vi "运维调试_采配水.vi"() -> ()   [LabVIEW 2016, in "PLC.lvlib"]
uses:
  PLC.lvlib
  <vilib>/Plasmionique/MB Master/MB_Master/MB_Master.lvclass
  <vilib>/Utility/miscctls.llb/LVPointTypeDef.ctl
  <vilib>/Plasmionique/MB Master/MB_Master_Serial/MB_Master_Serial.lvclass
  C:/Program Files (x86)/National Instruments/LabVIEW 2016/vi.lib/Plasmionique/MB Master/MB_Master/MB_Master.lvclass
  <vilib>/Instr/_visa.llb/VISA Configure Serial Port (Instr).vi
  <vilib>/Plasmionique/MB Master/MB Master.lvlib
panel:
  in  "看门狗启用":bool
  out "R123":i16 caption="看门狗设置"
  out "R56":i16 caption="看门狗计时器"
  in  "释放串口":bool
  out "R122":i16 caption="二级自来水清洗时间"
  out "R121":i16 caption="一级自来水清洗时间"
  out "R120":i16 caption="过滤自来水清洗时间"
  out "清洗次数":u16
  out "R119":i16 caption="多参数启动延时"
  out "当前启动泵号":u16(ring) items=["1号泵", "2号泵"]
  out "R116":i16 caption="储水时间"
  in  "R113":u16(ring) caption="水箱储水水体" items=["自来水", "水样"]
  out "R112":i16 caption="二级水样池进样超时"
  in  "R111":u16(ring) caption="采配水型号" items=["常规版本", "高配版本"]
  out "数值 19":dbl
  out "数值 18":dbl
  out "数值 17":dbl
  out "数值 16":dbl
  out "数值 15":dbl
  out "数值 14":dbl
  out "数值 13":dbl
  out "数值 12":dbl
  out "数值 11":dbl
  out "数值 10":dbl
  out "数值 9":dbl
  out "数值 8":dbl
  out "数值 7":dbl
  out "数值 6":dbl
  out "数值 5":dbl
  out "数值 4":dbl
  out "数值 3":dbl
  out "数值 2":dbl
  out "数值":dbl
  in  "R118":u16(ring) caption="是否启用质控" items=["不启用质控", "启用质控"]
  out "压力传感器":dbl format="%#.2f"
  out "R110":i16 caption="过滤装置排液时间"
  in  "M4":bool
  in  "M3":bool
  in  "V13":bool
  in  "V12":bool
  in  "V1-R":bool
  in  "V1-G":bool
  in  "V11":bool
  in  "V10":bool
  in  "V9":bool
  in  "V8":bool
  in  "V7-R":bool
  in  "V7-G":bool
  out "X2":bool caption="X1"
  out "采配水版本号":string
  out "R117":i16 caption="清洗频次设定"
  out "通讯故障":bool
  in  "R100":u16(ring) caption="采水泵工作模式" items=["泵1单泵单管路", "泵2单泵单管路", "潜水泵双泵双管路", "自吸泵双泵双管路"]
  out "X11":bool caption="自来水检测_WA"
  out "X10":bool caption="废液报警_WLA"
  out "X9":bool caption="泵2过载报警_KM2"
  out "X8":bool caption="泵1过载报警_KM1"
  out "X7":bool caption="断电检测_DD"
  out "X6":bool caption="门禁开关_MJ"
  out "X5":bool caption="烟雾检测_YW"
  out "X4":bool caption="浸水检测_SJ"
  out "X3":bool caption="水流开关_JY"
  out "X1":bool
  out "X0":bool caption="采样池液位开关_YE1"
  out "R109":i16 caption="外部反冲洗时间"
  out "集成报警信息":string
  out "R108":i16 caption="进样超时时间"
  out "R107":i16 caption="进气时间"
  out "R106":i16 caption="排液时间"
  out "R105":i16 caption="配水时间"
  out "R104":i16 caption="过滤次数"
  out "R103":i16 caption="过滤配水时间"
  out "R102":i16 caption="静置沉淀时间"
  out "R101":i16 caption="管路润洗时间"
  out "R2":i16
  out "R1":i16
  out "多列列表框":i32(listbox)
  in  "V6":bool
  in  "V5":bool
  in  "V4":bool
  in  "V3":bool
  in  "V2":bool
  in  "M2":bool
  in  "M1":bool
  in  "返回":bool
  in  "参数设置":bool
  in  "单步启动":bool
  in  "启动":bool
  in  "停止":bool
  # "流程计时："
  # "s"
  # "压力传感器："
  # "MPa"
  # "二级液位开关低_Y2FD"
  # "二级液位开关高_YF2H"
  # "看门狗设置"
  # "S"
  # "S"
  # "S"
  # "S"
  # "S"
  # "S"
  # "S"
  # "S"
  # "次"
  # "S"
  # "S"
  # "S"
  # "S"
  # "S"
  # "S"
  # "单步计时："
  # "s"
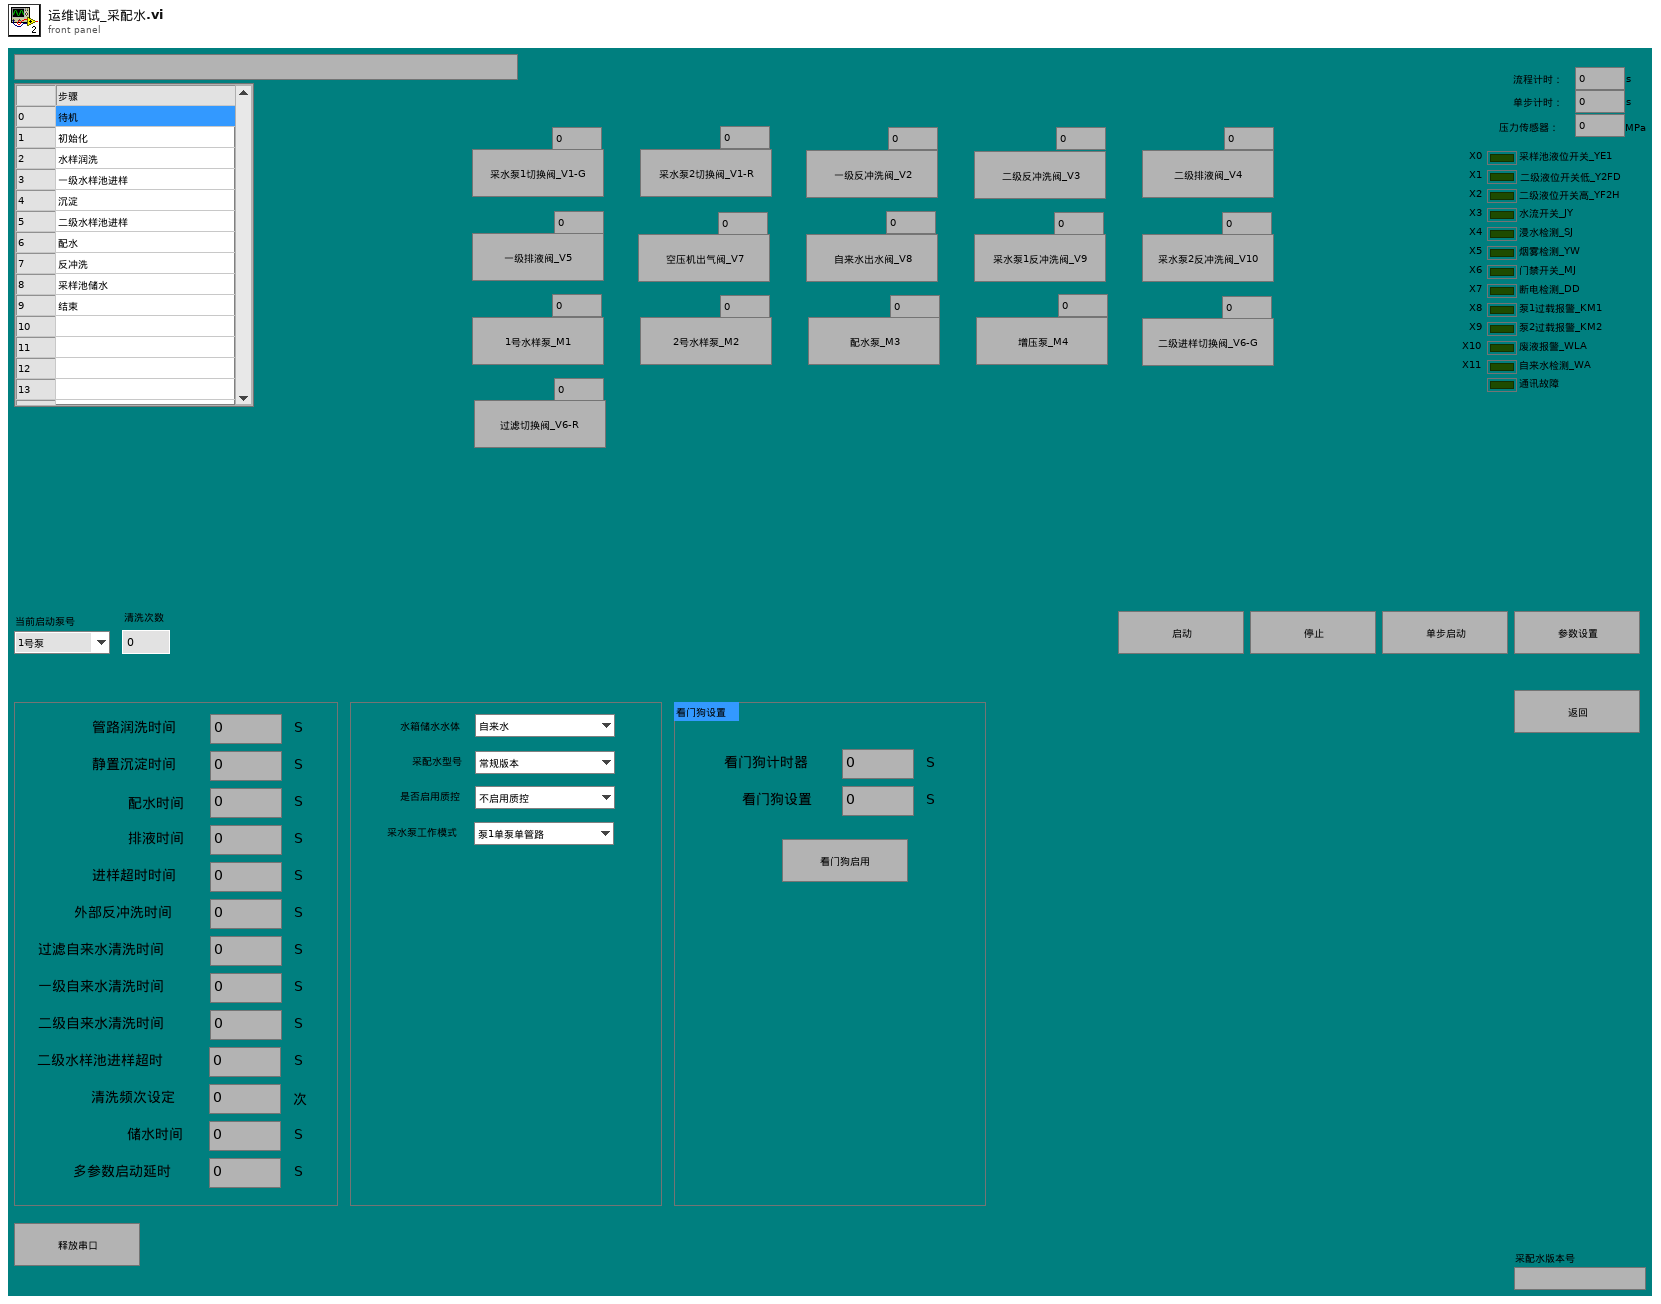
[diagram p1: front panel]
types:
  T1 = typedef "LVPointTypeDef.ctl" = cluster{"Horizontal":i16, "Vertical":i16}
  T2 = cluster{"命令":string, "数据":cluster{"starting address":u16, "holding register value":u16}}
  T3 = cluster{"时间标识":timestamp, "设备":string, "日志信息":string}
  T4 = cluster{"R0":i16, "R1":i16, "R2":i16, "R3":i16, "R4":i16, "R5":i16, "R6":i16, "R7":i16, "R8":i16, "R9":i16, "R10":i16, "R11":i16, "R12":i16, "R13":i16, "R14":i16, "R15":i16, "R16":i16, "R17":i16, "R18":i16, "R19":i16, "R20":i16, "R21":i16, "R22":i16, "R23":i16, "R24":i16, "R25":i16, "R26":i16, "R27":i16, "R28":i16, "R29":i16, "R30":i16, "R31":i16, "R32":i16, "R33":i16, "R34":i16, "R35":i16, "R36":i16, "R37":i16, "R38":i16, "R39":i16, "R40":i16, "R41":i16, "R42":i16, "R43":i16, "R44":i16, "R45":i16, "R46":i16, "R47":i16, "R48":i16, "R49":i16, "R50":i16, "R51":i16, "R52":i16, "R53":i16, "R54":i16, "R55":i16, "R56":i16}
  T5 = cluster{"seconds since 1Jan1904":timestamp, "table输入":string, string, "table输入":string}
  T6 = cluster{"时间标识":timestamp, "设备":string, "日志信息":string, "流程参数":string}
  T7 = cluster{"命令":string, cluster{"starting address":u16, "holding register value":u16}}
  T8 = cluster{"CODCr":cluster{"启动测量模式":cluster{"测量模式":enum16{"水样测量", "标样核查", "零点核查", "跨度核查", "空白测试", "加标回收", "平行样", "校零", "校标"}}, "确定按钮":bool}, "参数启用":cluster{"多参数":bool, "CODMn":bool, "总磷总氮":bool, "氨氮":bool, "CODcr":bool}}
  T9 = enum16{"水样测量", "标样核查", "零点核查", "跨度核查", "空白测试", "加标回收", "平行样", "校零", "校标"}
  T10 = cluster{"命令":string, "数据":cluster{"starting address":u16, "holding register values":u16[]}}
  T11 = cluster{"命令":string, "data":cluster{"starting address":u16, "coil values":bool[]}}
  T12 = cluster{"多参数":bool, "CODMn":bool, "总磷总氮":bool, "氨氮":bool, "CODcr":bool}
  T13 = enum32{"Bad", "Idle", "Run top level", "Running"}
  T14 = cluster{"baud rate (bps)":u32, "stop bits":u16, "parity":u16, "flow control":u16, "timeout":u32, "retries":i32}
  T15 = cluster{"starting address":u16, "holding register values":u16[]}
  T16 = cluster{"starting address":u16, "holding register value":u16}
  T17 = cluster{"starting address":u16, "coil values":bool[]}
  T18 = cluster{"Registers[0]":u16, "Registers[1]":u16, "Registers[2]":u16, "Registers[3]":u16, "Registers[4]":u16, "Registers[5]":u16, "Registers[6]":u16, "Registers[7]":u16, "Registers[8]":u16, "Registers[9]":u16, "Registers[10]":u16, "Registers[11]":u16, "Registers[12]":u16, "Registers[13]":u16, "Registers[14]":u16, "Registers[15]":u16, "Registers[16]":u16, "Registers[17]":u16, "Registers[18]":u16, "Registers[19]":u16, "Registers[20]":u16, "Registers[21]":u16, "Registers[22]":u16, "Registers[23]":u16, "Registers[24]":u16, "Registers[25]":u16, "Registers[26]":u16, "Registers[27]":u16, "Registers[28]":u16, "Registers[29]":u16, "Registers[30]":u16, "Registers[31]":u16, "Registers[32]":u16, "Registers[33]":u16, "Registers[34]":u16, "Registers[35]":u16, "Registers[36]":u16, "Registers[37]":u16, "Registers[38]":u16, "Registers[39]":u16, "Registers[40]":u16, "Registers[41]":u16, "Registers[42]":u16, "Registers[43]":u16, "Registers[44]":u16, "Registers[45]":u16, "Registers[46]":u16, "Registers[47]":u16, "Registers[48]":u16, "Registers[49]":u16, "Registers[50]":u16, "Registers[51]":u16, "Registers[52]":u16, "Registers[53]":u16, "Registers[54]":u16, "Registers[55]":u16, "Registers[56]":u16}
  T19 = cluster{"Registers[0]":u16, "Registers[1]":u16, "Registers[2]":u16, "Registers[3]":u16, "Registers[4]":u16, "Registers[5]":u16}
  T20 = cluster{"Registers[0]":u16, "Registers[1]":u16, "Registers[2]":u16, "Registers[3]":u16, "Registers[4]":u16, "Registers[5]":u16, "Registers[6]":u16, "Registers[7]":u16, "Registers[8]":u16, "Registers[9]":u16, "Registers[10]":u16, "Registers[11]":u16, "Registers[12]":u16, "Registers[13]":u16, "Registers[14]":u16, "Registers[15]":u16, "Registers[16]":u16, "Registers[17]":u16, "Registers[18]":u16, "Registers[19]":u16, "Registers[20]":u16, "Registers[21]":u16, "Registers[22]":u16, "Registers[23]":u16}
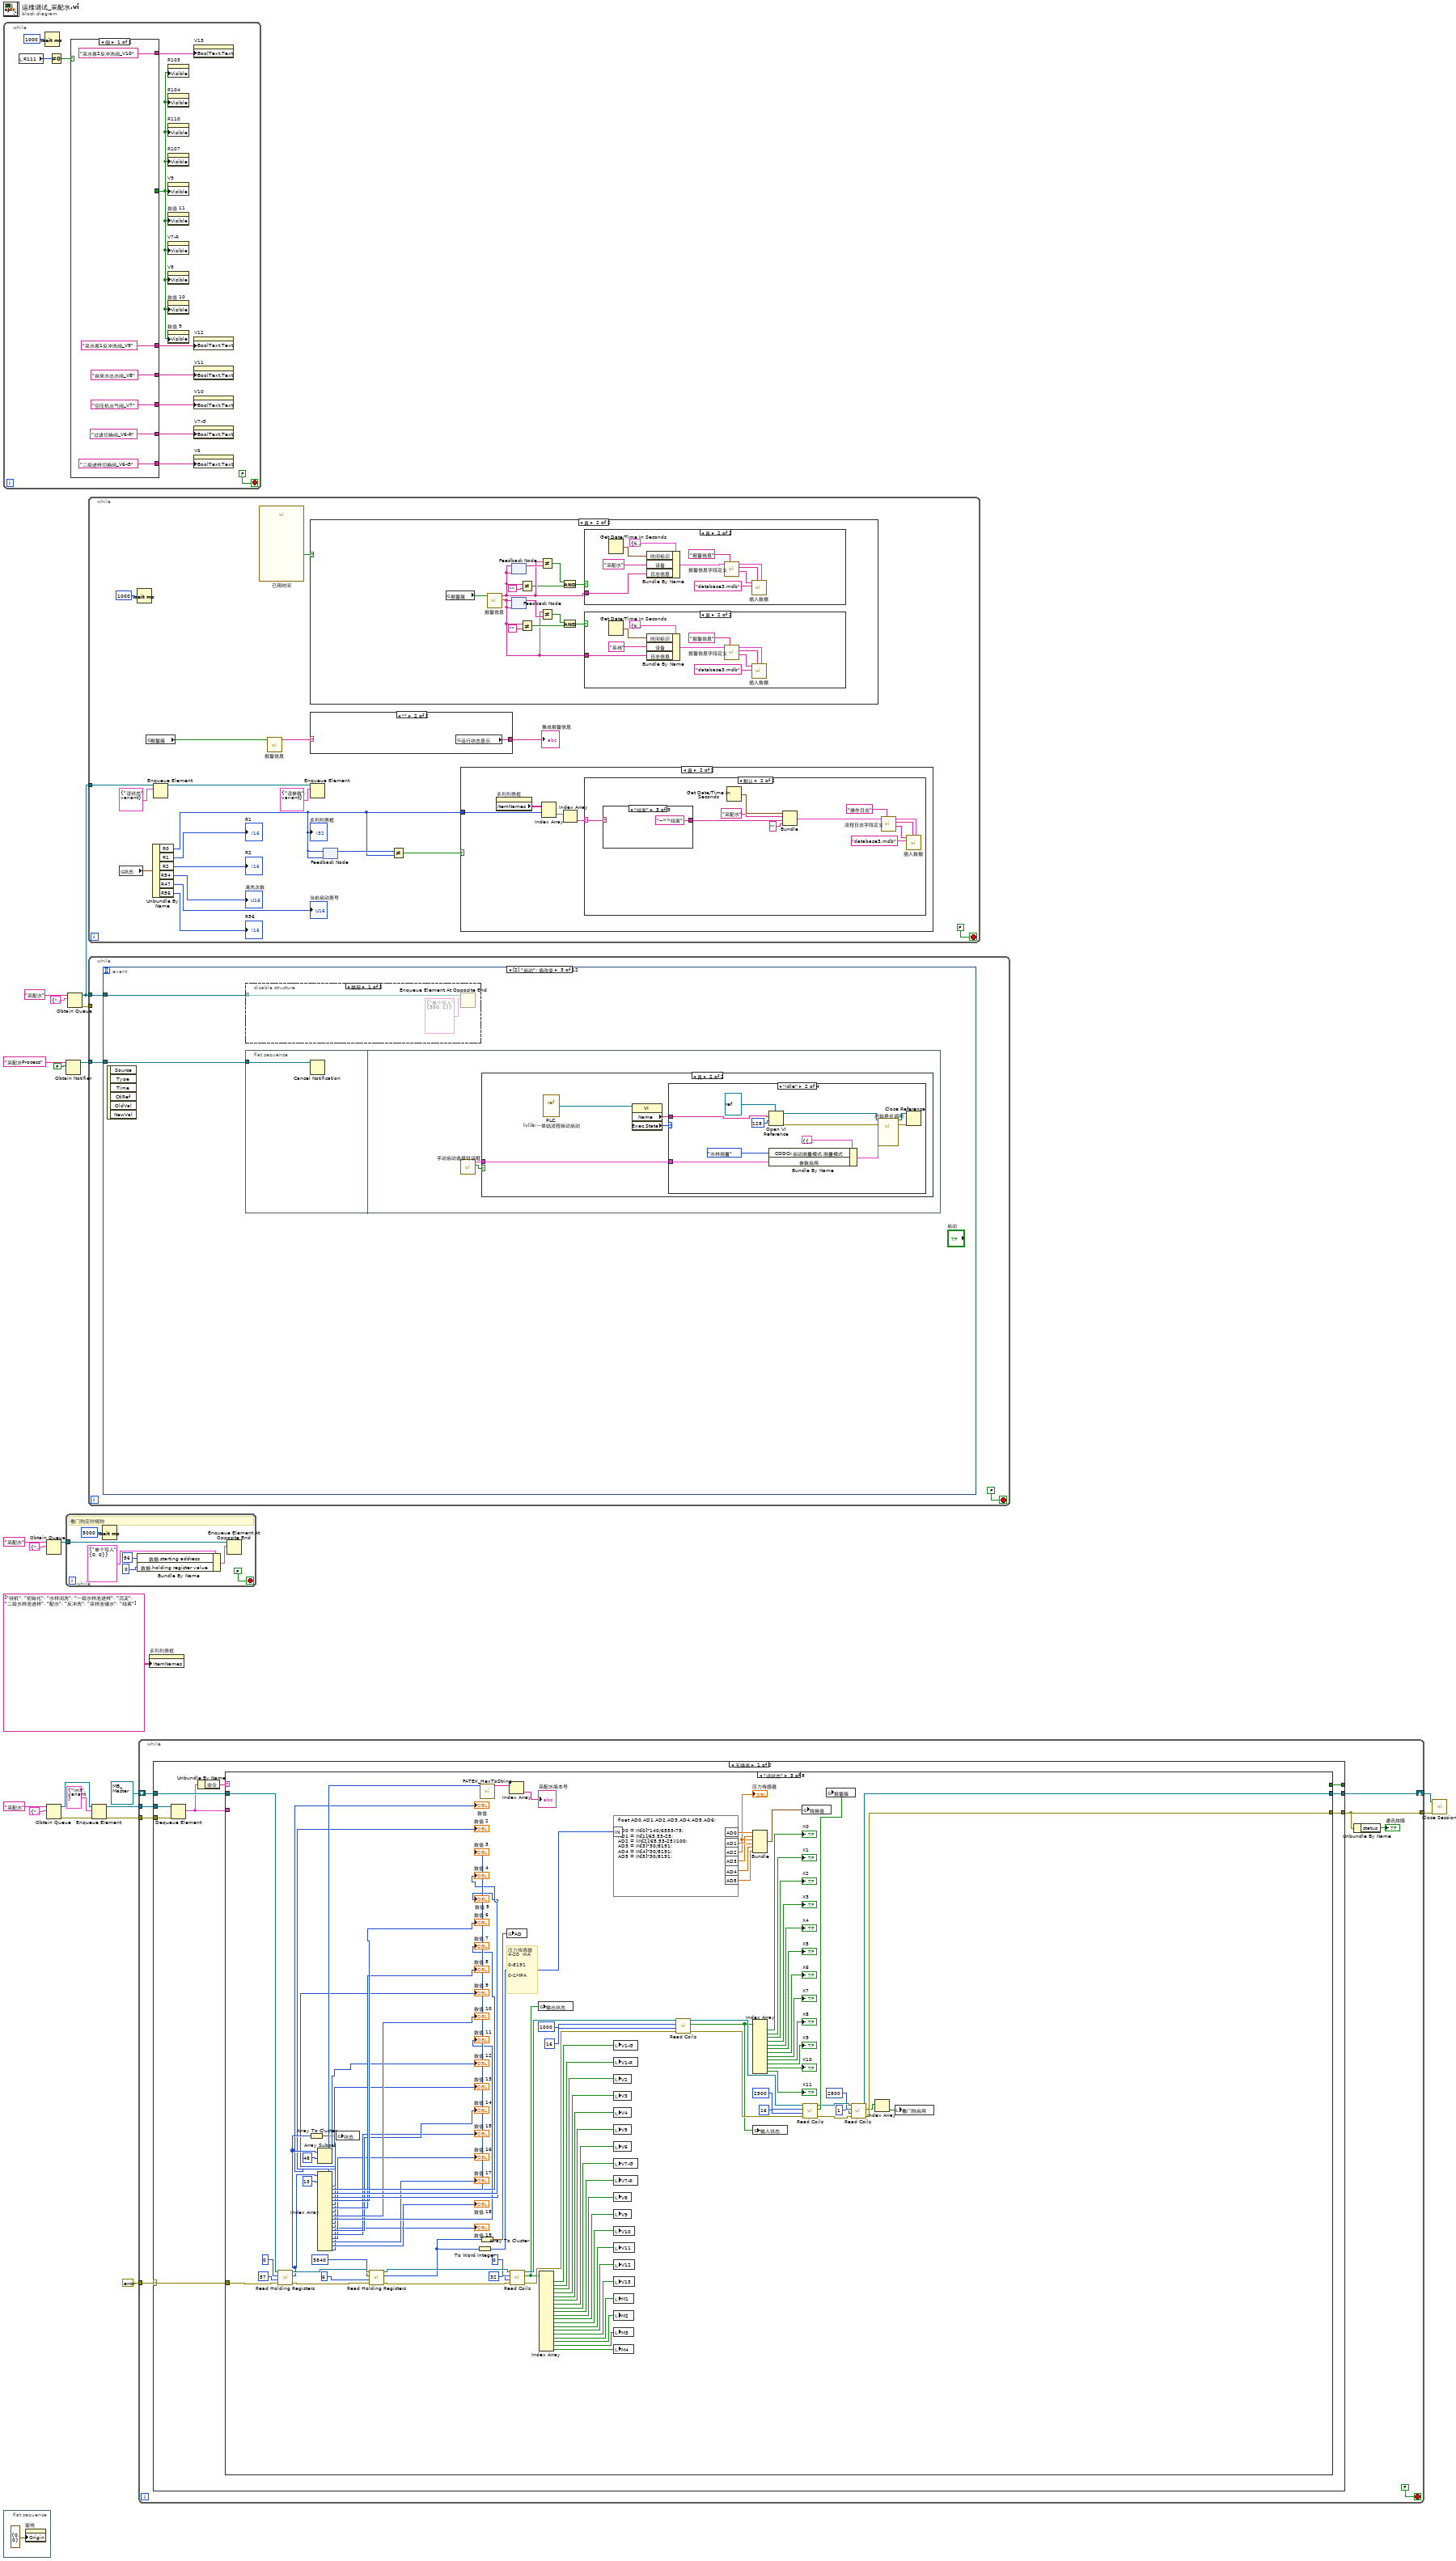
[diagram p0: block diagram]
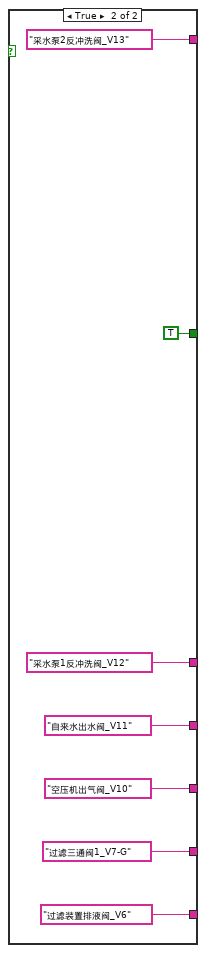
[diagram p2: hidden frame]
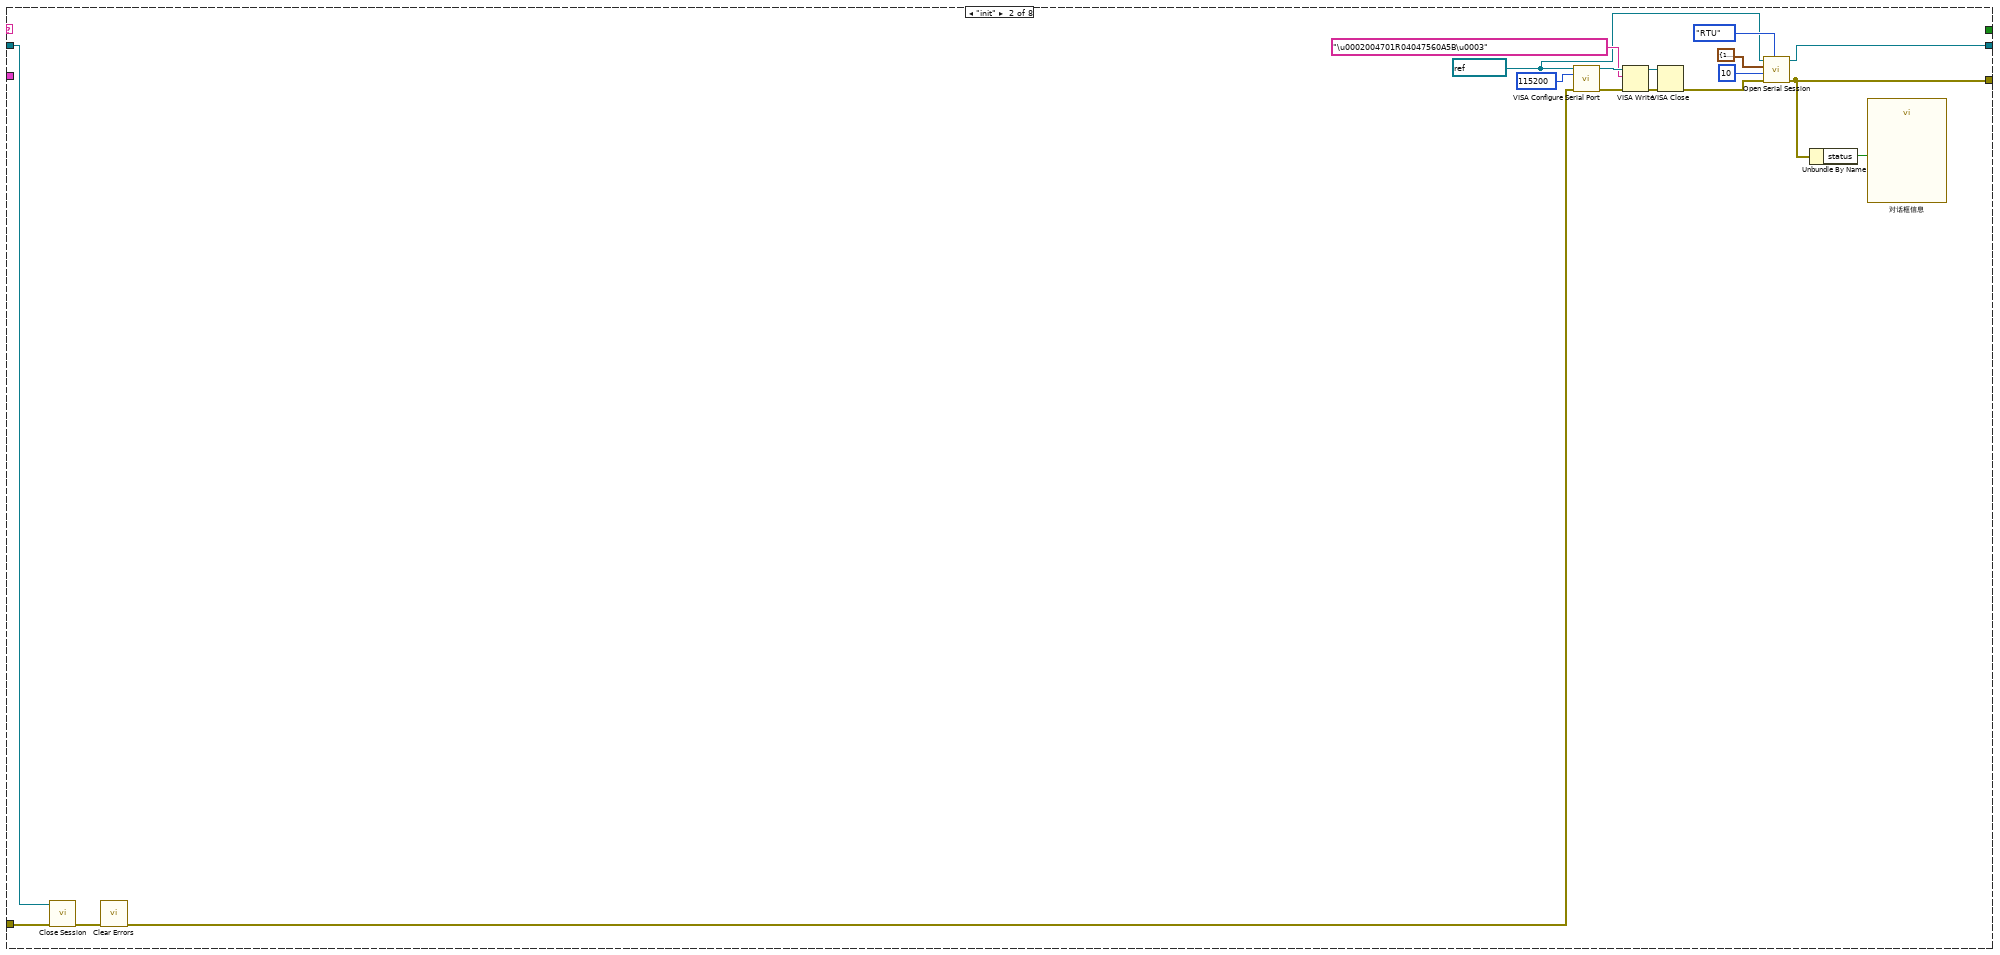
[diagram p4: hidden frame]
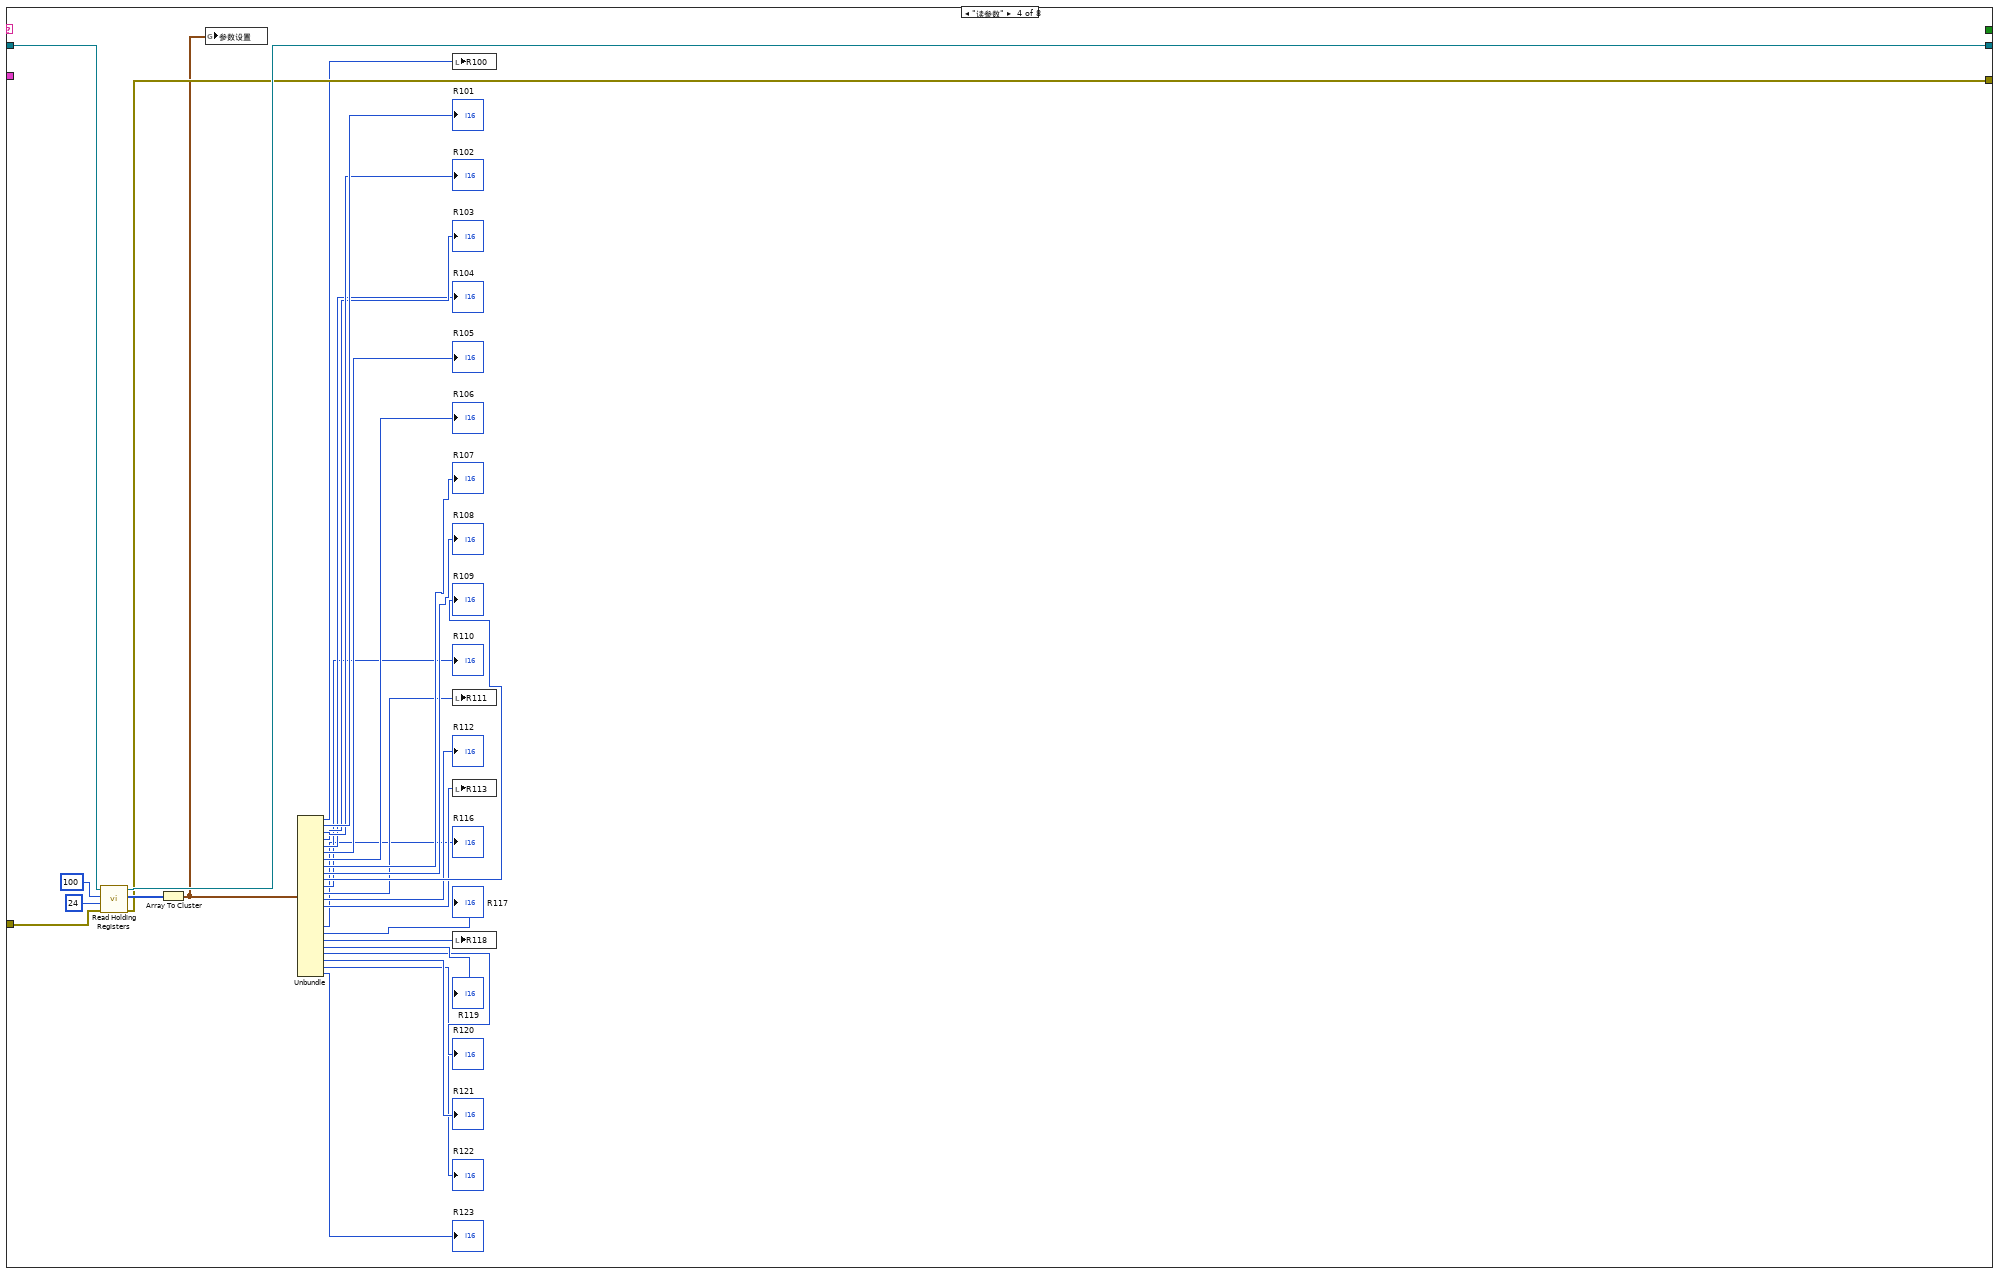
[diagram p5: hidden frame]
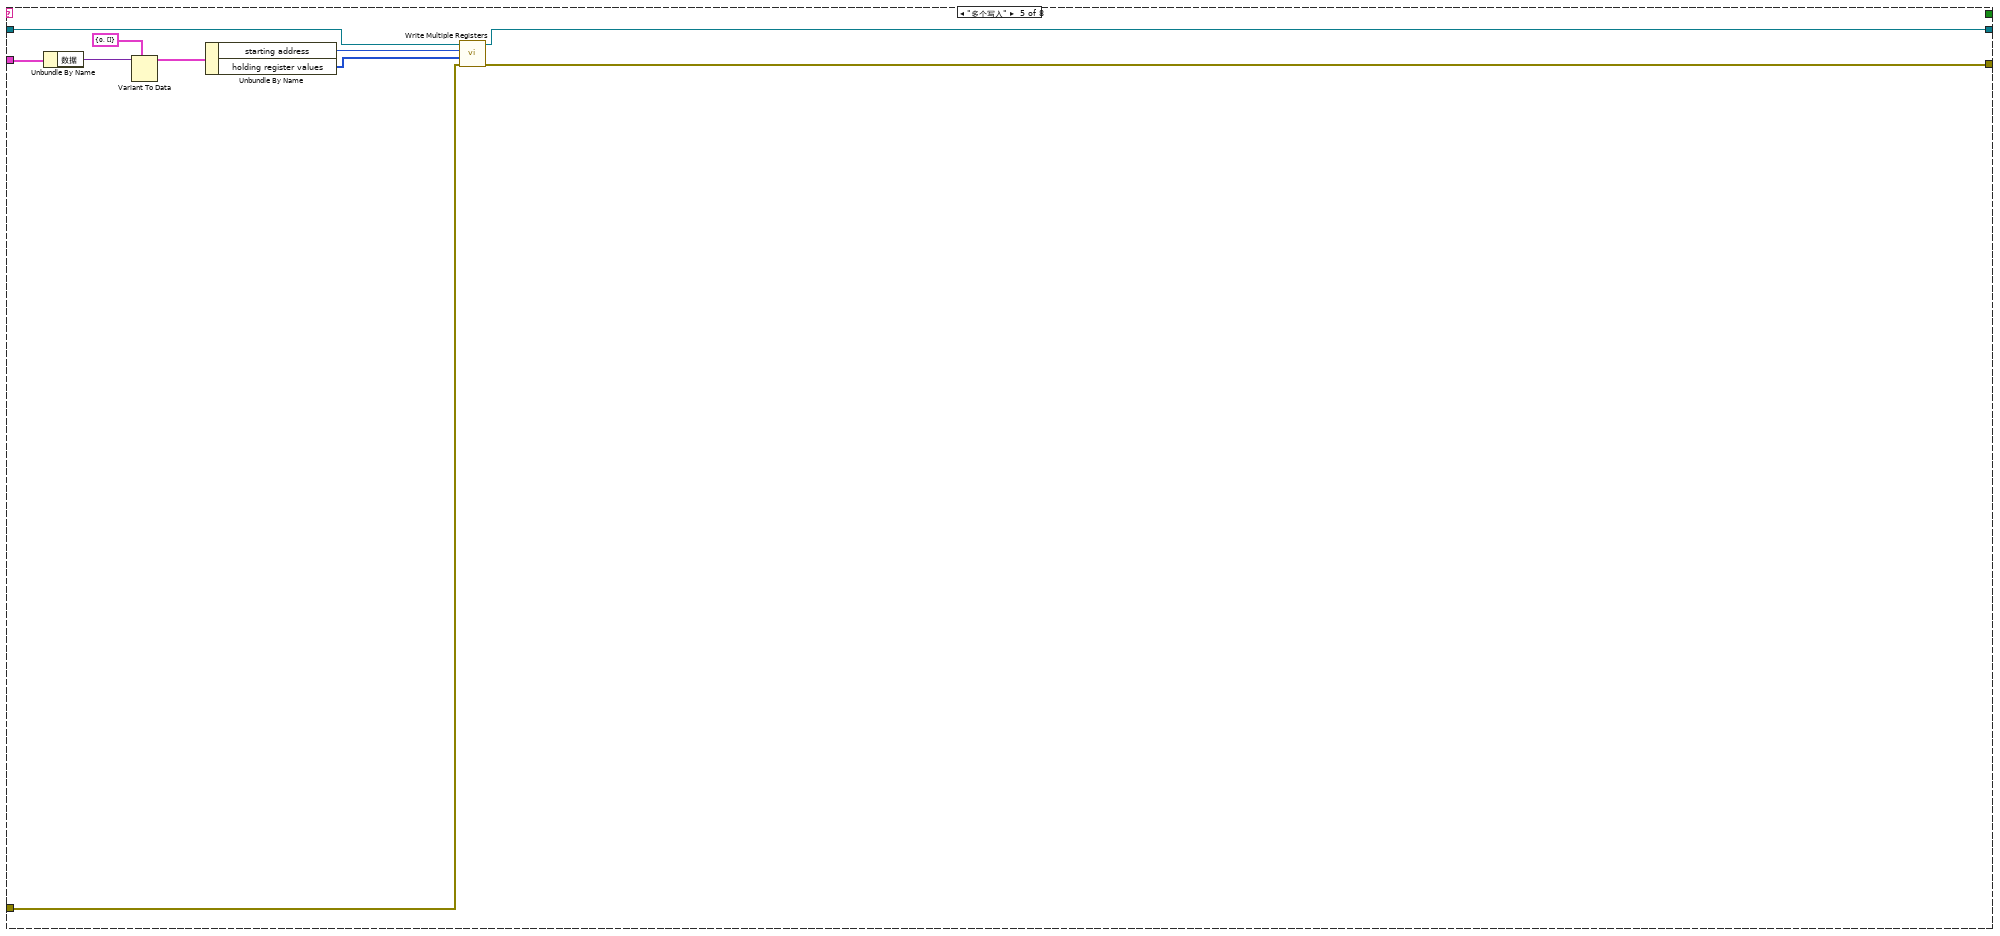
[diagram p6: hidden frame]
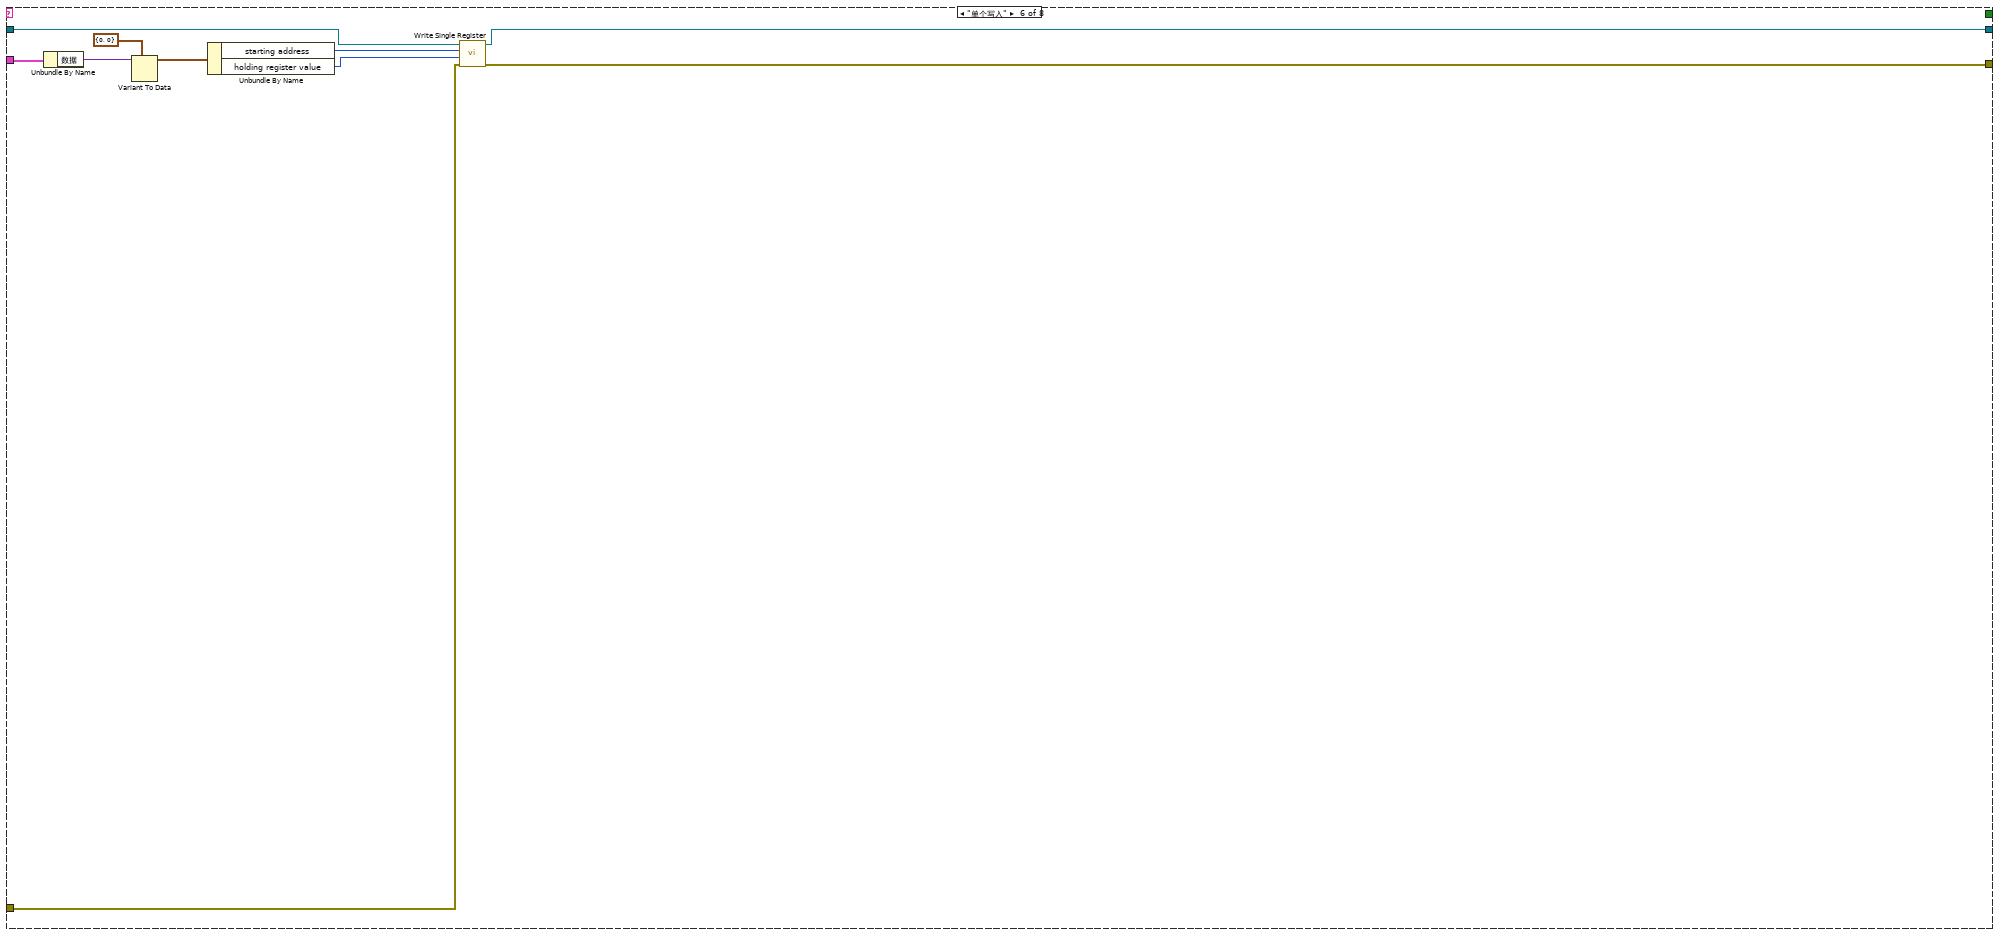
[diagram p7: hidden frame]
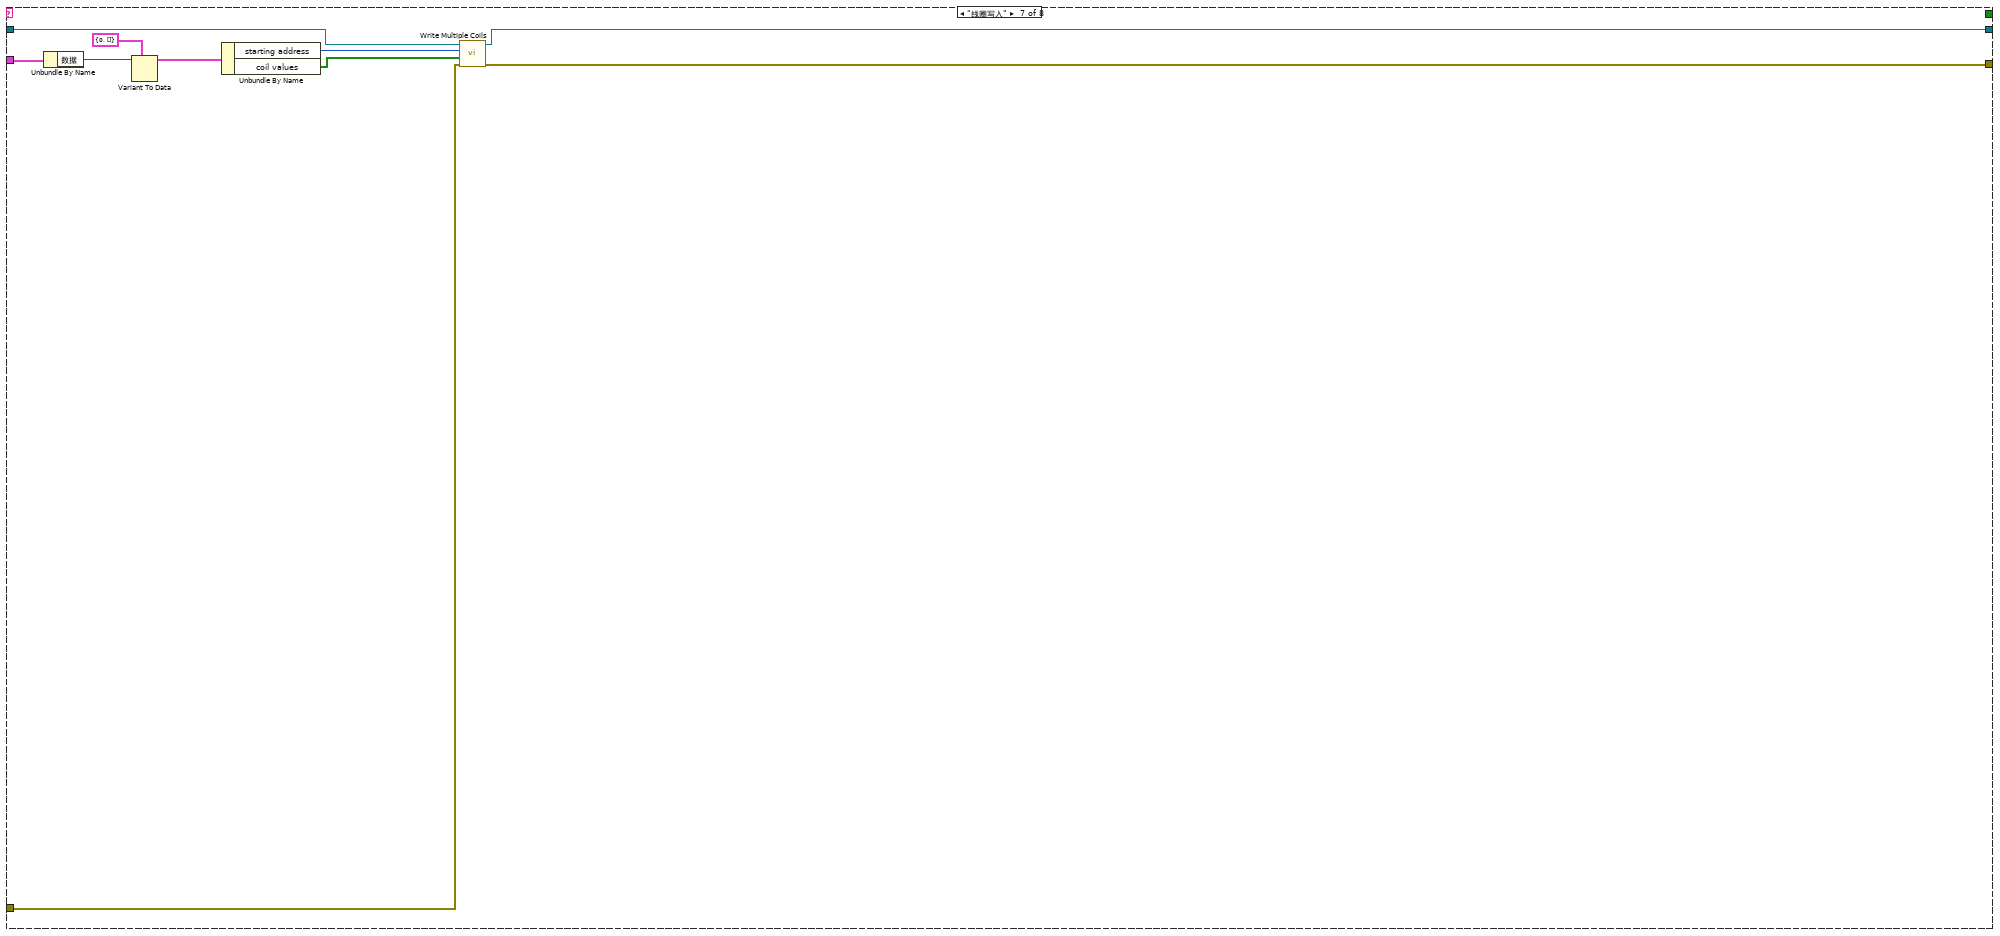
[diagram p8: hidden frame]
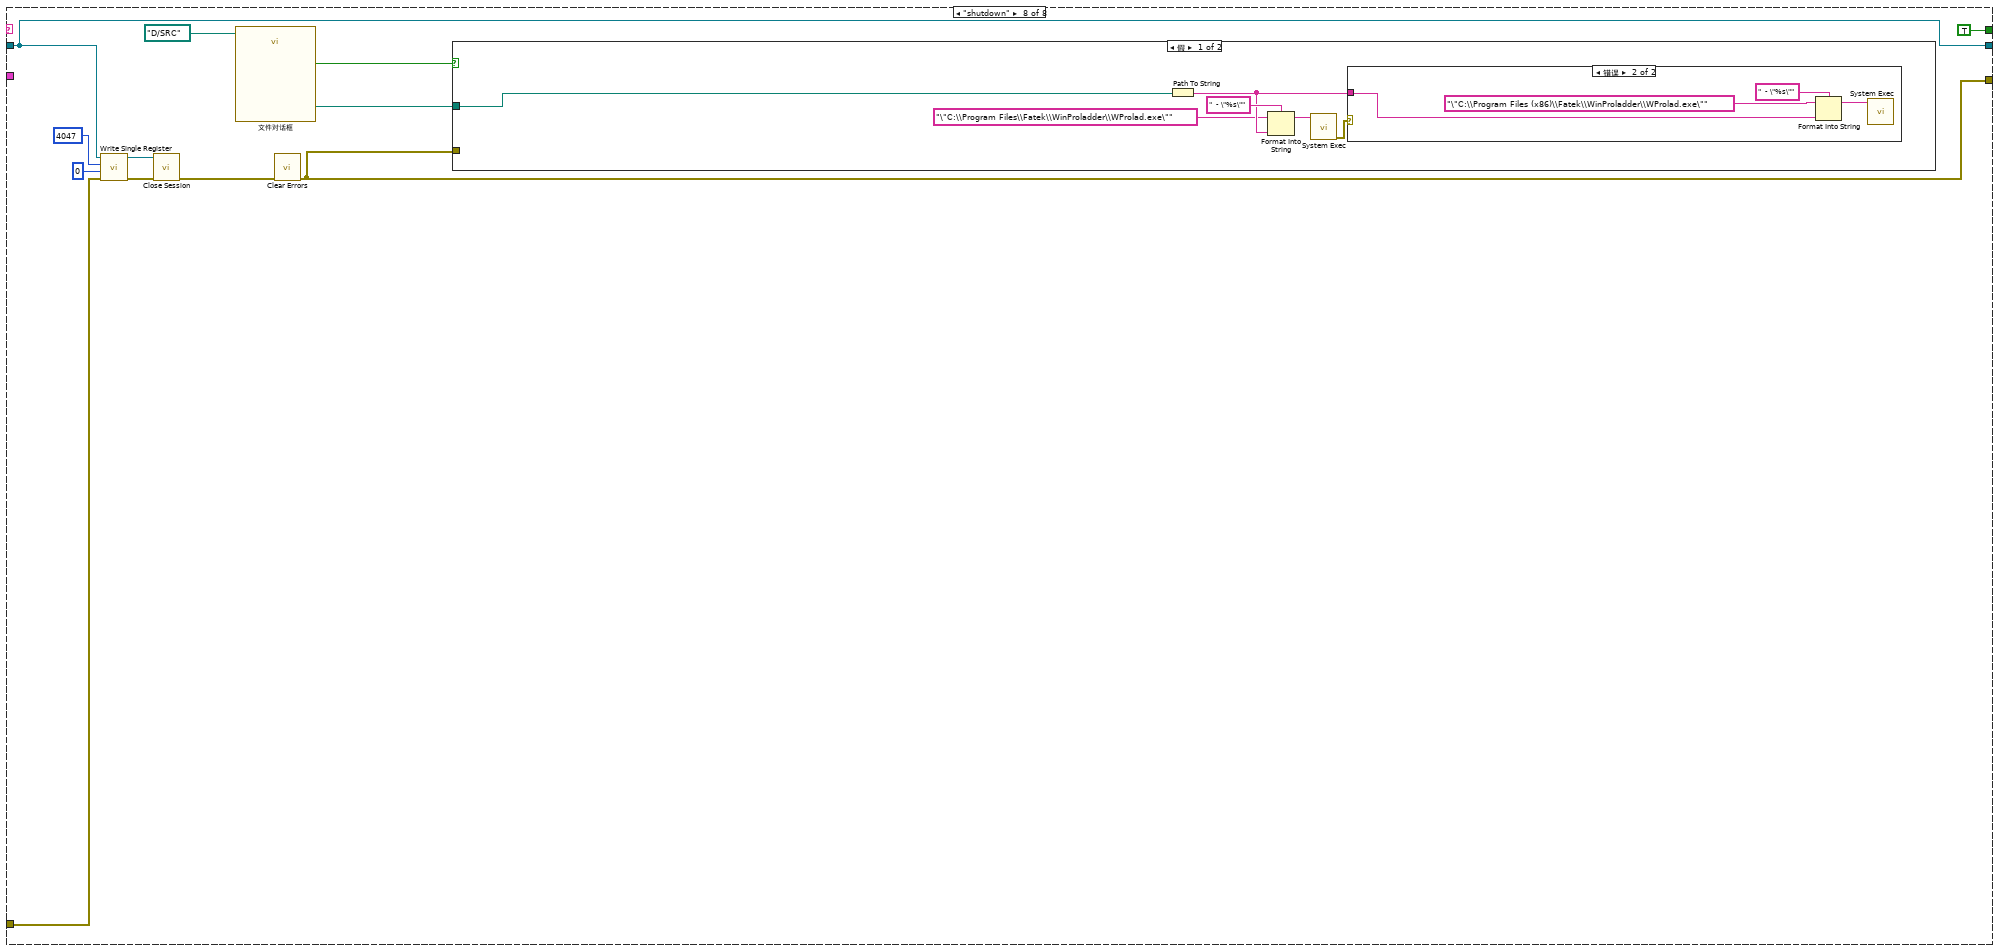
[diagram p9: hidden frame]
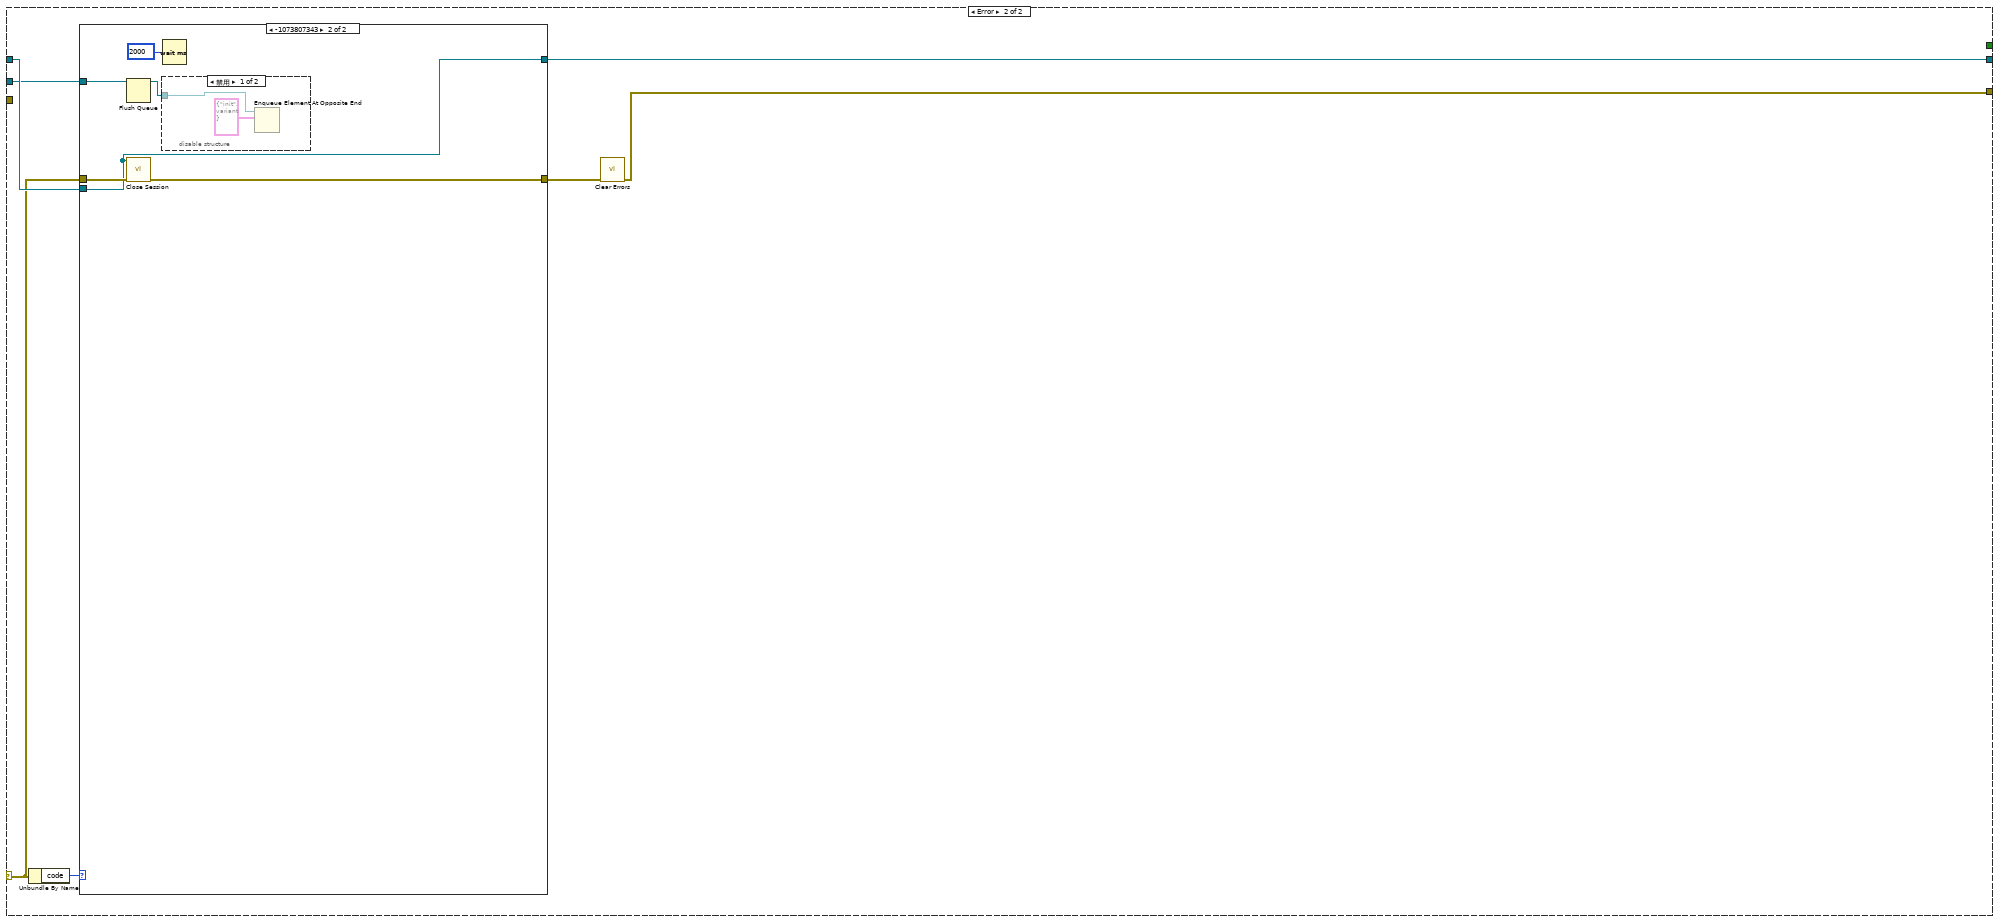
[diagram p12: hidden frame]
diagram:
  n1 = while {
    stop <- FALSE stop-if-true
    n2 = local read "R111"() -> (w32:u16)
    n3 = Wait (ms)(milliseconds to wait=u32 1000 ("等待时间（毫秒）")) -> ()  [unwired: 1 out]
    n4 = Not Equal To 0?(x=w32) -> (x != 0?=w31:bool)
    n5 = case shown="假" w31 {
      tunnel: [_ TRUE ("可见")] -> w30
      tunnel: ["二级进样切换阀_V6-G" ("布尔文本.文本") "过滤装置排液阀_V6" ("布尔文本.文本")] -> w28
      tunnel: ["过滤切换阀_V6-R" ("布尔文本.文本") "过滤三通阀1_V7-G" ("布尔文本.文本")] -> w27
      tunnel: ["空压机出气阀_V7" ("布尔文本.文本") "空压机出气阀_V10" ("布尔文本.文本")] -> w26
      tunnel: ["自来水出水阀_V8" ("布尔文本.文本") "自来水出水阀_V11" ("布尔文本.文本")] -> w25
      tunnel: ["采水泵1反冲洗阀_V9" ("布尔文本.文本") "采水泵1反冲洗阀_V12" ("布尔文本.文本")] -> w24
      tunnel: ["采水泵2反冲洗阀_V10" ("布尔文本.文本") "采水泵2反冲洗阀_V13" ("布尔文本.文本")] -> w23
      frame False {
      }
      frame True {
      }
    }
    n6 = property on="R103" class="DigNum (严格)"("Visible"=w30) -> ()  [unwired: 2 in, 2 out]
    n7 = property on="R104" class="DigNum (严格)"("Visible"=w30) -> ()  [unwired: 2 in, 2 out]
    n8 = property on="R110" class="DigNum (严格)"("Visible"=w30) -> ()  [unwired: 2 in, 2 out]
    n9 = property on="R107" class="DigNum (严格)"("Visible"=w30) -> ()  [unwired: 2 in, 2 out]
    n10 = property on="V9" class="Bool (严格)"("Visible"=w30) -> ()  [unwired: 2 in, 2 out]
    n11 = property on="数值 11" class="DigNum (严格)"("Visible"=w30) -> ()  [unwired: 2 in, 2 out]
    n12 = property on="V7-R" class="Bool (严格)"("Visible"=w30) -> ()  [unwired: 2 in, 2 out]
    n13 = property on="V8" class="Bool (严格)"("Visible"=w30) -> ()  [unwired: 2 in, 2 out]
    n14 = property on="数值 10" class="DigNum (严格)"("Visible"=w30) -> ()  [unwired: 2 in, 2 out]
    n15 = property on="数值 9" class="DigNum (严格)"("Visible"=w30) -> ()  [unwired: 2 in, 2 out]
    n16 = property on="V13" class="Bool (严格)"("BoolText.Text"=w23) -> ()  [unwired: 2 in, 2 out]
    n17 = property on="V12" class="Bool (严格)"("BoolText.Text"=w24) -> ()  [unwired: 2 in, 2 out]
    n18 = property on="V11" class="Bool (严格)"("BoolText.Text"=w25) -> ()  [unwired: 2 in, 2 out]
    n19 = property on="V10" class="Bool (严格)"("BoolText.Text"=w26) -> ()  [unwired: 2 in, 2 out]
    n20 = property on="V7-G" class="Bool (严格)"("BoolText.Text"=w27) -> ()  [unwired: 2 in, 2 out]
    n21 = property on="V6" class="Bool (严格)"("BoolText.Text"=w28) -> ()  [unwired: 2 in, 2 out]
  }
  n22 = flat-sequence {
    frame #0 {
      n23 = property on="窗格" class="Pane"("Origin"=T1 {"Horizontal"=0, "Vertical"=0} ("原点")) -> ()  [unwired: 2 in, 2 out]
    }
  }
  n24 = Obtain Queue(name (unnamed)="采配水" ("名称（未命名）"), element data type=cluster{"命令":string, "数据":variant} {"命令"="", "数据"=variant}) -> (queue out=w1:refnum<queue>)  [unwired: 3 in, 2 out]
  n25 = Obtain Queue(name (unnamed)="采配水" ("名称（未命名）"), element data type=cluster{"命令":string, "数据":variant} {"命令"="", "数据"=variant}) -> (queue out=w12:refnum<queue>, error out=w11:errorcluster)  [unwired: 3 in, 1 out]
  n26 = Obtain Notifier(name (unnamed)="采配水Process" ("名称（未命名）"), notification data type=FALSE) -> (notifier out=w15:refnum<notifier>)  [unwired: 2 in, 2 out]
  n27 = while {
    tunnel: w1 -> [w52]
    stop <- FALSE stop-if-true
    # "看门狗定时喂狗"
    n28 = Wait (ms)(milliseconds to wait=u32 5000 ("等待时间（毫秒）")) -> ()  [unwired: 1 out]
    n29 = Bundle By Name(cluster=T2 {"命令"="单个写入", "数据"={"starting address"=0, "holding register value"=0}} ("元素"), "数据.starting address"=u16 56, "数据.holding register value"=u16 0) -> (w53:T2)
    n30 = Enqueue Element At Opposite End(queue=w52, element=w53) -> ()  [unwired: 2 in, 3 out]
  }
  n31 = Obtain Queue(name (unnamed)="采配水" ("名称（未命名）"), element data type=cluster{"命令":string, "数据":variant} {"命令"="", "数据"=variant}) -> (queue out=w19:refnum<queue>, error out=w20:errorcluster)  [unwired: 3 in, 1 out]
  n32 = while {
    tunnel: w19 -> [w72]
    stop <- FALSE stop-if-true
    n33 = global read "采配水全局变量.vi" "状态"() -> (w70:T4)
    n34 = Wait (ms)(milliseconds to wait=u32 1000 ("等待时间（毫秒）")) -> ()  [unwired: 1 out]
    n35 = global read "采配水全局变量.vi" "报警簇"() -> (w66:bool[])
    n36 = Unbundle By Name(w70) -> ("R0"=w59:i16, "R1"=→"R1":i16, "R2"=→"R2":i16, "R54"=→"清洗次数":i16, "R47"=→"当前启动泵号":i16, "R56"=→"R56":i16)
    "多列列表框" <- w59
    n37 = Enqueue Element(queue=w72, element=cluster{"命令":string, "数据":variant} {"命令"="读状态", "数据"=variant} ("元素")) -> (queue out=w61:refnum<queue>)  [unwired: 2 in, 2 out]
    n38 = call "已用时间"() -> ("Time has Elapsed"=w64:bool)  [unwired: 12 in, 7 out]
    n39 = call "报警信息.vi"("报警簇"=w66) -> ("采配水报警信息"=w58:string)  [unwired: 9 in, 1 out]
    n40 = case shown="真" w64 {
      frame False {
      }
      frame True {
        n41 = global read "采配水全局变量.vi" "报警簇"() -> (w86:bool[])
        n42 = call "报警信息.vi"("报警簇"=w86) -> ("系统报警信息"=w75:string, "采配水报警信息"=w82:string)  [unwired: 9 in]
        n43 = feedback #1(w82) -> (w85:string)
        n44 = feedback-in #1(w82) -> ()
        n45 = feedback #2(w75) -> (w76:string)
        n46 = feedback-in #2(w75) -> ()
        n47 = Not Equal?(x=w82, y="") -> (x != y?=w80:bool)
        n48 = Not Equal?(x=w75, y="") -> (x != y?=w79:bool)
        n49 = Not Equal?(x=w82, y=w85) -> (x != y?=w84:bool)
        n50 = Not Equal?(x=w75, y=w76) -> (x != y?=w77:bool)
        n51 = And(x=w84, y=w80) -> (x .and. y?=w83:bool)
        n52 = And(x=w77, y=w79) -> (x .and. y?=w74:bool)
        n53 = case shown="真" w83 {
          tunnel: w82 -> [_ w97]
          frame False {
          }
          frame True {
            n54 = Get Date/Time In Seconds() -> (seconds since 1Jan1904=w99:timestamp)
            n55 = Bundle By Name(cluster=T3 {"时间标识"=timestamp(0 s since 1904-01-01), "设备"="", "日志信息"=""} ("data in"), "时间标识"=w99, "设备"="采配水", "日志信息"=w97) -> (w100:T3)
            n56 = call "报警信息字段定义.vi"("table输入"="报警信息", "data in"=w100) -> ("table输出"=w104:string, "columns"=w105:string[], "data out"=w106:T3)  [unwired: 7 in]
            n57 = call "插入数据.vi"("data"=w106, "columns"=w105, "database"="database3.mdb", "table"=w104) -> ()  [unwired: 7 in, 1 out]
          }
        }
        n58 = case shown="真" w74 {
          tunnel: w75 -> [_ w87]
          frame False {
          }
          frame True {
            n59 = Get Date/Time In Seconds() -> (seconds since 1Jan1904=w89:timestamp)
            n60 = Bundle By Name(cluster=T3 {"时间标识"=timestamp(0 s since 1904-01-01), "设备"="", "日志信息"=""} ("data in"), "时间标识"=w89, "设备"="系统", "日志信息"=w87) -> (w90:T3)
            n61 = call "报警信息字段定义.vi"("table输入"="报警信息", "data in"=w90) -> ("table输出"=w94:string, "columns"=w95:string[], "data out"=w96:T3)  [unwired: 7 in]
            n62 = call "插入数据.vi"("data"=w96, "columns"=w95, "database"="database3.mdb", "table"=w94) -> ()  [unwired: 7 in, 1 out]
          }
        }
      }
    }
    n63 = case shown="\"\"" w58 {
      selector: w58 -> [w107 _]
      tunnel: [w107 w108] -> w65
      frame Default {
      }
      frame "" {
        n64 = global read "采配水全局变量.vi" "运行状态显示"() -> (w108:string)
      }
    }
    "集成报警信息" <- w65
    n65 = Enqueue Element(queue=w61, element=cluster{"命令":string, "数据":variant} {"命令"="读参数", "数据"=variant} ("元素")) -> ()  [unwired: 2 in, 3 out]
    n66 = feedback-in #3(w59) -> ()
    n67 = feedback #3(w59) -> (w60:i16)
    n68 = Not Equal?(x=w60, y=w59) -> (x != y?=w67:bool)
    n69 = case shown="真" w67 {
      tunnel: w59 -> [_ w111]
      frame False {
      }
      frame True {
        n70 = property on="多列列表框" class="MCListbox (严格)"() -> ("ItemNames"=w112:string[][])  [unwired: 2 in, 2 out]
        n71 = Index Array(array=w112, index (row)=w111) -> (element=w110:string[])  [unwired: 1 in]
        n72 = Index Array(array=w110) -> (element=w109:string)  [unwired: 1 in]
        n73 = case shown="默认" w109 {
          selector: w109 -> [_ w114]
          frame "待机" {
          }
          frame Default {
            n74 = case shown="\"结束\"" w114 {
              selector: w114 -> [w124 _ _]
              tunnel: [w124 "-->>初始化" "-->>结束"] -> w113
              frame Default {
              }
              frame "初始化" {
              }
              frame "结束" {
              }
            }
            n75 = Get Date/Time In Seconds() -> (seconds since 1Jan1904=w118:timestamp)
            n76 = Bundle("seconds since 1Jan1904"=w118, "table输入"="采配水", w113, "table输入"="") -> (w116:T5)  [unwired: 1 in]
            n77 = call "流程日志字段定义.vi"("table输入"="操作日志", "data in"=w116) -> ("table输出"=w121:string, "columns"=w122:string[], "data out"=w123:T6)  [unwired: 7 in]
            n78 = call "插入数据.vi"("data"=w123, "columns"=w122, "database"="database3.mdb", "table"=w121) -> ()  [unwired: 7 in, 1 out]
          }
        }
      }
    }
  }
  n79 = while {
    tunnel: w19 -> [w128]
    tunnel: w20 -> [_]
    tunnel: w15 -> [w127]
    stop <- FALSE stop-if-true
    n80 = event shown="[2] \"启动\": 值改变" {
      selector: _ -> [_ _ _ _ _ _ _ _ _ _ _ _]
      dyn-events: _ -> [_ _ _ _ _ _ _ _ _ _ _ _]
      timeout: _ -> [_ _ _ _ _ _ _ _ _ _ _ _]
      tunnel: w128 -> [_ w132 w135 w160 w179 w189 _ _ _ w221 w224 w230]
      tunnel: w127 -> [_ w131 w134 _ _ _ _ _ _ _ _ _]
      event Timeout {
        n81 = event-data() -> ()  [unwired: 1 in, 3 out]
      }
      event "停止": Value Change {
        n82 = event-data() -> ()  [unwired: 1 in, 6 out]
        n83 = Send Notification(notification=TRUE ("通知"), notifier=w131) -> ()  [unwired: 1 in, 2 out]
        n84 = Enqueue Element At Opposite End(queue=w132, element=T7 {"命令"="单个写入", {"starting address"=300, "holding register value"=2}} ("元素")) -> ()  [unwired: 2 in, 3 out]
      }
      event "启动": Value Change {
        n85 = event-data() -> ()  [unwired: 1 in, 6 out]
        n86 = disable-structure shown="禁用" {
          disable-tunnel: w135 -> [w156 _]
          frame Disabled {
            n87 = Enqueue Element At Opposite End(queue=w156, element=T7 {"命令"="单个写入", {"starting address"=300, "holding register value"=1}} ("元素")) -> ()  [unwired: 2 in, 3 out]
          }
          frame Enabled {
          }
        }
        n88 = flat-sequence {
          tunnel: w134 -> [w136]
          frame #0 {
            n89 = Cancel Notification(0:w136) -> ()  [unwired: 1 in, 3 out]
          }
          frame #1 {
            n90 = call "手动启动选择对话框.vi"() -> ("确定"=w138:bool, "参数启用"=w137:T12)  [unwired: 10 in]
            n91 = case shown="真" w138 {
              tunnel: w137 -> [_ w139]
              frame False {
              }
              frame True {
                n92 = vi-ref "PLC.lvlib:一体站流程自动启动.vi"() -> (w142:refnum<vi>)
                n93 = property class="VI"(reference=w142) -> ("Name"=w141:string, "Exec.State"=w140:T13)  [unwired: 1 in, 2 out]
                n94 = case shown="\"Idle\"" w140 {
                  tunnel: w141 -> [_ w153 _ _]
                  tunnel: w139 -> [_ w147 _ _]
                  frame "Bad", Default {
                  }
                  frame "Idle" {
                    n95 = Bundle By Name(cluster=T8 {"CODCr"={"启动测量模式"={"测量模式"=enum."水样测量"}, "确定按钮"=FALSE}, "参数启用"={"多参数"=FALSE, "CODMn"=FALSE, "总磷总氮"=FALSE, "氨氮"=FALSE, "CODcr"=FALSE}} ("参数"), "CODCr.启动测量模式.测量模式"=T9."水样测量", "参数启用"=w147) -> (w143:T8)
                    n96 = Open VI Reference(type specifier VI Refnum (for type only)=refnum<vi> refnum, vi path=w153, options=128 ("选项")) -> (vi reference=w151:refnum<vi>, error out=w149:errorcluster)  [unwired: 3 in]
                    n97 = call-by-ref "开始异步调用"(reference=w151, error in=w149, "参数"=w143) -> (reference out=w150:refnum<vi>, error out=w148:errorcluster)  [unwired: 11 in]
                    n98 = Close Reference(reference=w150, error in (no error)=w148) -> ()  [unwired: 1 out]
                  }
                  frame "Run top level" {
                  }
                  frame "Running" {
                    n99 = One Button Dialog(message="流程已启动，无需重复启动！" ("消息")) -> ()  [unwired: 1 in, 1 out]
                  }
                }
              }
            }
          }
        }
      }
      event "单步启动": Value Change {
        n100 = event-data() -> ()  [unwired: 1 in, 6 out]
        n101 = call "单步启动对话框.vi"() -> ("单步启动步骤输出"=w157:u16)  [unwired: 11 in]
        n102 = Bundle By Name(cluster=T2 {"命令"="单个写入", "数据"={"starting address"=301, "holding register value"=0}} ("元素"), "数据.holding register value"=w157) -> (w158:T2)
        n103 = Enqueue Element At Opposite End(queue=w160, element=w158) -> ()  [unwired: 2 in, 3 out]
      }
      event "R101", "R102", "R103", "R104", "R105", "R106", "R107", "R108", "R109", "R100", "R110", "R111", "R112", "R113": Value Change {
        n104 = event-data() -> ()  [unwired: 1 in, 6 out]
        n105 = local read "R101"() -> (w175:i16)
        n106 = local read "R102"() -> (w174:i16)
        n107 = local read "R103"() -> (w173:i16)
        n108 = local read "R104"() -> (w172:i16)
        n109 = local read "R105"() -> (w171:i16)
        n110 = local read "R106"() -> (w170:i16)
        n111 = local read "R107"() -> (w169:i16)
        n112 = local read "R108"() -> (w168:i16)
        n113 = local read "R109"() -> (w166:i16)
        n114 = local read "R110"() -> (w165:i16)
        n115 = local read "R112"() -> (w162:i16)
        n116 = Build Array("R100", w175, w174, w173, w172, w171, w170, w169, w168, w166, w165, "R111", w162, "R113") -> (w164:u16[])
        n117 = Bundle By Name(cluster=T10 {"命令"="多个写入", "数据"={"starting address"=0, "holding register values"=[]}} ("元素"), "数据.starting address"=u16 100, "数据.holding register values"=w164) -> (w176:T10)
        n118 = Enqueue Element At Opposite End(queue=w179, element=w176) -> ()  [unwired: 2 in, 3 out]
      }
      event "R116", "R117", "R118", "R119", "R120", "R121", "R122", "R123": Value Change {
        n119 = event-data() -> ()  [unwired: 1 in, 6 out]
        n120 = local read "R116"() -> (w187:i16)
        n121 = local read "R117"() -> (w186:i16)
        n122 = local read "R119"() -> (w184:i16)
        n123 = local read "R120"() -> (w183:i16)
        n124 = local read "R121"() -> (w182:i16)
        n125 = local read "R122"() -> (w181:i16)
        n126 = local read "R123"() -> (w180:i16)
        n127 = Build Array(w187, w186, "R118", w184, w183, w182, w181, w180) -> (w188:u16[])
        n128 = Bundle By Name(cluster=T10 {"命令"="多个写入", "数据"={"starting address"=0, "holding register values"=[]}} ("元素"), "数据.starting address"=u16 116, "数据.holding register values"=w188) -> (w190:T10)
        n129 = Enqueue Element At Opposite End(queue=w189, element=w190) -> ()  [unwired: 2 in, 3 out]
      }
      event "R101", "R102", "R103", "R104", "R105", "R106", "R107", "R108", "R109", "R117", "R110", "R116", "R112", "R119", "R120", "R121", "R122", "R123": Mouse Down {
        n130 = event-data() -> ("CtlRef"=w196:refnum<vi>)  [unwired: 1 in, 7 out]
        n131 = property class="DigNum (严格)"(reference=w196) -> (reference out=w194:refnum<vi>, "Value"=w195:i16)  [unwired: 1 in, 1 out]
        n132 = call "数字键盘.vi"("OldNumber"=w195) -> ("NewNumber"=w193:sgl)
        n133 = property class="DigNum (严格)"(reference=w194, "Val(Sgnl)"=w193) -> ()  [unwired: 1 in, 2 out]
      }
      event "参数设置": Value Change {
        n134 = event-data() -> ()  [unwired: 1 in, 6 out]
        n135 = property on="窗格" class="Pane"("Origin"=T1 {"Horizontal"=0, "Vertical"=628} ("原点")) -> ()  [unwired: 2 in, 2 out]
      }
      event "返回": Value Change {
        n136 = event-data() -> ()  [unwired: 1 in, 6 out]
        n137 = property on="窗格" class="Pane"("Origin"=T1 {"Horizontal"=0, "Vertical"=0} ("原点")) -> ()  [unwired: 2 in, 2 out]
      }
      event "M1", "M2", "V2", "V3", "V4", "V5", "V6", "V7-G", "V7-R", "V8", "V9", "V10", "V11", "V1-G", "V1-R", "V12", "V13", "M4", "M3": Value Change {
        n138 = event-data() -> ()  [unwired: 1 in, 6 out]
        n139 = Build Array("V1-G", "V1-R", "V2", "V3", "V4", "V5", "V6", "V7-G", "V7-R", "V8", "V9", "V10", "V11", "V12", "V13", "M1", "M2", "M3", "M4") -> (w214:bool[])
        n140 = Bundle By Name(cluster=T11 {"命令"="线圈写入", "data"={"starting address"=2400, "coil values"=[]}} ("元素"), "data.coil values"=w214) -> (w215:T11)
        n141 = Enqueue Element(queue=w221, element=w215) -> ()  [unwired: 2 in, 3 out]
      }
      event "看门狗启用": Value Change {
        n142 = event-data() -> ("NewVal"=w223:bool)  [unwired: 1 in, 5 out]
        n143 = Build Array(w223) -> (w222:bool[])
        n144 = Bundle By Name(cluster=T11 {"命令"="线圈写入", "data"={"starting address"=2800, "coil values"=[]}} ("元素"), "data.coil values"=w222) -> (w225:T11)
        n145 = Enqueue Element(queue=w224, element=w225) -> ()  [unwired: 2 in, 3 out]
      }
      event "释放串口": Value Change {
        n146 = event-data() -> ("NewVal"=w227:bool)  [unwired: 1 in, 5 out]
        n147 = case shown="真" w227 {
          tunnel: [cluster{"命令":string, "数据":variant} {"命令"="init", "数据"=variant} ("元素") w234] -> w229
          frame False {
          }
          frame True {
            n148 = Two Button Dialog(message="警告，非专业人士请勿进行此操作！！！\n请确认是否释放串口？" ("消息")) -> (T button?=w233:bool)  [unwired: 2 in]
            n149 = case shown="真" w233 {
              tunnel: [_ cluster{"命令":string, "数据":variant} {"命令"="shutdown", "数据"=variant} ("元素")] -> w234
              frame False {
                n150 = local write "释放串口"(FALSE ("释放串口")) -> ()
              }
              frame True {
              }
            }
          }
        }
        n151 = Flush Queue(queue=w230) -> (queue out=w228:refnum<queue>)  [unwired: 1 in, 2 out]
        n152 = Enqueue Element(queue=w228, element=w229) -> ()  [unwired: 2 in, 3 out]
      }
    }
  }
  n153 = Enqueue Element(queue=w12, element=cluster{"命令":string, "数据":variant} {"命令"="init", "数据"=variant} ("元素"), error in (no error)=w11) -> (queue out=w7:refnum<queue>, error out=w9:errorcluster)  [unwired: 1 in, 1 out]
  n154 = while {
    tunnel: w7 -> [w241]
    tunnel: w9 -> [w240]
    shift-right: [w244] -> w4
    shift-left: refnum<class "MB_Master.lvclass"> refnum ("MB session in") -> [w243]
    tunnel: errorcluster {"status"=FALSE, "code"=0, "source"=""} ("error out") -> [w242]
    tunnel: [w239] -> w5
    stop <- FALSE stop-if-true
    n155 = case shown="无错误" w242 {
      selector: w242 -> [w250 w458]
      tunnel: [w253 w457] -> w244
      tunnel: w243 -> [w252 w459]
      tunnel: [w251 w455] -> w239
      tunnel: w241 -> [w247 w454]
      tunnel: w240 -> [w246 _]
      tunnel: [w248 _] -> _
      frame No Error {
        n156 = Dequeue Element(queue=w247, error in (no error)=w246) -> (element=w245:cluster{"命令":string, "数据":variant})  [unwired: 1 in, 3 out]
        n157 = Unbundle By Name(w245) -> ("命令"=w249:string)
        n158 = case shown="\"读状态\"" w249 {
          tunnel: [w255 w268 w280 w396 w408 w418 w428 w441] -> w253
          tunnel: w252 -> [w255 w270 w361 w401 w411 w421 w431 w441]
          tunnel: [w254 w269 w278 w395 w409 w419 w429 w432] -> w251
          tunnel: w250 -> [w254 w272 w364 w400 w410 w420 w430 w437]
          tunnel: [_ _ _ _ _ _ _ TRUE] -> w248
          tunnel: w245 -> [_ _ _ _ w407 w417 w427 _]
          frame "idle", Default {
          }
          frame "init" {
            w259 = refnum<visa-resource-name> "COM3" ("VISA resource name")
            n159 = call-dynamic "Close Session.vi"("error in (no error)"=w272, "MB session in"=w270) -> ("error out"=w271:errorcluster)  [unwired: 9 in]
            n160 = call <vilib>:"Clear Errors.vi"("error in (no error)"=w271) -> ("error out"=w257:errorcluster)  [unwired: 5 in, 1 out]
            n161 = call-poly "VISA Configure Serial Port"("VISA resource name"=w259, "baud rate (9600)"=u32 115200, "error in (no error)"=w257) -> ("VISA resource name out"=w264:refnum<visa-resource-name>, "error out"=w263:errorcluster)  [unwired: 11 in]
            n162 = VISA Write(VISA resource name=w264, write buffer="\u0002004701R04047560A5B\u0003" ("写入缓冲区"), error in (no error)=w263) -> (VISA resource name out=w262:refnum<visa-resource-name>, error out=w261:errorcluster)  [unwired: 1 out]
            n163 = VISA Close(VISA resource name=w262, error in (no error)=w261) -> (error out=w256:errorcluster)
            n164 = call <vilib>:"Open Serial Session.vi"("Mode (RTU)"=enum16{"RTU", "ASCII"}."RTU", "Error in"=w256, "Slave ID"=u8 10, "Serial Config"=T14 {"baud rate (bps)"=115200, "stop bits"=10, "parity"=0, "flow control"=0, "timeout"=500, "retries"=1}, "VISA Resource"=w259) -> ("Error out"=w269:errorcluster, "MB_Serial session"=w268:refnum<class "MB_Master_Serial.lvclass">)  [unwired: 5 in]
            n165 = Unbundle By Name(w269) -> ("status"=w273:bool)
            n166 = call "对话框信息"("Enable"=w273) -> ()  [unwired: 9 in, 2 out]
          }
          frame "读状态" {
            # "压力传感器\n4-20  mA \n \n0-8191\n\n0-1MPA"
            n167 = call <vilib>:"Read Holding Registers.vi"("error in (no error)"=w364, "quantity"=u16 57 ("number of holding registers"), "starting address"=u16 0, "MB session in"=w361) -> ("error out"=w359:errorcluster, "Registers"=w303:u16[], "MB session out"=w360:refnum<class "MB_Master.lvclass">)  [unwired: 5 in]
            n168 = Array To Cluster(array=w303) -> (cluster=w282:T18)
            n169 = Array Subset(array=w303, index=48 ("索引")) -> (w329:u16[])  [unwired: 1 in]
            n170 = Index Array(array=w303, index #1=13 ("索引")) -> (element #1=→"数值":u16, element #2=→"数值 2":u16, element #3=→"数值 3":u16, element #4=→"数值 4":u16, element #5=→"数值 5":u16, element #6=→"数值 6":u16, element #7=→"数值 7":u16, element #8=→"数值 8":u16, element #9=→"数值 9":u16, element #10=→"数值 10":u16, element #11=→"数值 11":u16, element #12=→"数值 12":u16, element #13=→"数值 13":u16, element #14=→"数值 14":u16, element #15=→"数值 15":u16, element #16=→"数值 16":u16, element #17=→"数值 17":u16, element #18=→"数值 18":u16, element #19=→"数值 19":u16)  [unwired: 18 in]
            n171 = global write "采配水全局变量.vi" "状态"(w282) -> ()
            n172 = call <vilib>:"Read Holding Registers.vi"("error in (no error)"=w359, "quantity"=u16 6 ("number of holding registers"), "starting address"=u16 3840, "MB session in"=w360) -> ("error out"=w355:errorcluster, "Registers"=w332:u16[], "MB session out"=w356:refnum<class "MB_Master.lvclass">)  [unwired: 5 in]
            n173 = To Word Integer(number=w332) -> (16bit integer=w331:i16[])
            n174 = call "FATEK_HexToString.vi"("数组"=w329) -> ("STRING"=w328:string[])  [unwired: 10 in]
            n175 = Array To Cluster(array=w332) -> (cluster=w371:T19)
            n176 = global write "采配水全局变量.vi" "AD"(w371) -> ()
            n177 = Index Array(array=w328) -> (element=→"采配水版本号":string)  [unwired: 1 in]
            n178 = call <vilib>:"Read Coils.vi"("error in (no error)"=w355, "quantity"=u16 32 ("number of coils"), "starting address"=u16 0, "MB session in"=w356) -> ("error out"=w351:errorcluster, "Coils"=w336:bool[], "MB session out"=w352:refnum<class "MB_Master.lvclass">)  [unwired: 5 in]
            n179 = global write "采配水全局变量.vi" "输出状态"(w336) -> ()
            n180 = Index Array(array=w336) -> (element #1=w310:bool, element #2=w326:bool, element #3=w325:bool, element #4=w324:bool, element #5=w323:bool, element #6=w322:bool, element #7=w321:bool, element #8=w317:bool, element #9=w316:bool, element #10=w315:bool, element #11=w314:bool, element #12=w313:bool, element #13=w312:bool, element #14=w309:bool, element #15=w308:bool, element #16=w307:bool, element #17=w306:bool, element #18=w305:bool, element #19=w304:bool)  [unwired: 19 in]
            n181 = formula code="float AD0,AD1,AD2,AD3,AD4,AD5,AD6;\n\nAD0 = IN[0]*140/6553-75;\nAD1 = IN[1]/65.53-25;\nAD2 = (IN[2]/65.53-25)/100;\nAD3 = IN[3]*30/8191;\nAD4 = IN[4]*30/8191;\nAD5 = IN[5]*30/8191;"("IN"=w331) -> ("AD0"=w369:dbl, "AD1"=w368:dbl, "AD2"=w311:dbl, "AD3"=w367:dbl, "AD4"=w366:dbl, "AD5"=w365:dbl)
            "压力传感器" <- w311
            n182 = local write "V1-G"(w310) -> ()
            n183 = local write "V1-R"(w326) -> ()
            n184 = local write "V2"(w325) -> ()
            n185 = local write "V3"(w324) -> ()
            n186 = local write "V4"(w323) -> ()
            n187 = local write "V5"(w322) -> ()
            n188 = local write "V6"(w321) -> ()
            n189 = local write "V7-G"(w317) -> ()
            n190 = local write "V7-R"(w316) -> ()
            n191 = local write "V8"(w315) -> ()
            n192 = local write "V9"(w314) -> ()
            n193 = local write "V10"(w313) -> ()
            n194 = local write "V11"(w312) -> ()
            n195 = local write "V12"(w309) -> ()
            n196 = local write "V13"(w308) -> ()
            n197 = local write "M1"(w307) -> ()
            n198 = local write "M2"(w306) -> ()
            n199 = local write "M3"(w305) -> ()
            n200 = local write "M4"(w304) -> ()
            n201 = call <vilib>:"Read Coils.vi"("error in (no error)"=w351, "quantity"=u16 16 ("number of coils"), "starting address"=u16 1000, "MB session in"=w352) -> ("error out"=w347:errorcluster, "Coils"=w343:bool[], "MB session out"=w348:refnum<class "MB_Master.lvclass">)  [unwired: 5 in]
            n202 = global write "采配水全局变量.vi" "输入状态"(w343) -> ()
            n203 = Bundle(w369, w368, w311, w367, w366, w365) -> (w370:cluster{dbl, dbl, dbl, dbl, dbl, dbl})  [unwired: 1 in]
            n204 = Index Array(array=w343) -> (element #1=→"X0":bool, element #2=→"X1":bool, element #3=→"X2":bool, element #4=→"X3":bool, element #5=→"X4":bool, element #6=→"X5":bool, element #7=→"X6":bool, element #8=→"X7":bool, element #9=→"X8":bool, element #10=→"X9":bool, element #11=→"X10":bool, element #12=→"X11":bool)  [unwired: 12 in]
            n205 = global write "采配水全局变量.vi" "转换值"(w370) -> ()
            n206 = call <vilib>:"Read Coils.vi"("error in (no error)"=w347, "quantity"=u16 16 ("number of coils"), "starting address"=u16 2500, "MB session in"=w348) -> ("error out"=w279:errorcluster, "Coils"=w344:bool[], "MB session out"=w281:refnum<class "MB_Master.lvclass">)  [unwired: 5 in]
            n207 = global write "采配水全局变量.vi" "报警簇"(w344) -> ()
            n208 = call <vilib>:"Read Coils.vi"("error in (no error)"=w279, "quantity"=u16 1, "starting address"=u16 2800, "MB session in"=w281) -> ("error out"=w278:errorcluster, "Coils"=w275:bool[], "MB session out"=w280:refnum<class "MB_Master.lvclass">)  [unwired: 5 in]
            n209 = Index Array(array=w275) -> (element=w274:bool)  [unwired: 1 in]
            n210 = local write "看门狗启用"(w274) -> ()
          }
          frame "读参数" {
            n211 = call <vilib>:"Read Holding Registers.vi"("error in (no error)"=w400, "quantity"=u16 24 ("number of holding registers"), "starting address"=u16 100, "MB session in"=w401) -> ("error out"=w395:errorcluster, "Registers"=w397:u16[], "MB session out"=w396:refnum<class "MB_Master.lvclass">)  [unwired: 5 in]
            n212 = Array To Cluster(array=w397) -> (cluster=w385:T20)
            n213 = global write "采配水全局变量.vi" "参数设置"(w385) -> ()
            n214 = Unbundle(w385) -> ("Registers[0]"=w384:u16, "Registers[1]"=→"R101":u16, "Registers[2]"=→"R102":u16, "Registers[3]"=→"R103":u16, "Registers[4]"=→"R104":u16, "Registers[5]"=→"R105":u16, "Registers[6]"=→"R106":u16, "Registers[7]"=→"R107":u16, "Registers[8]"=→"R108":u16, "Registers[9]"=→"R109":u16, "Registers[10]"=→"R110":u16, "Registers[11]"=w381:u16, "Registers[12]"=→"R112":u16, "Registers[13]"=w379:u16, "Registers[16]"=→"R116":u16, "Registers[17]"=→"R117":u16, "Registers[18]"=w377:u16, "Registers[19]"=→"R119":u16, "Registers[20]"=→"R120":u16, "Registers[21]"=→"R121":u16, "Registers[22]"=→"R122":u16, "Registers[23]"=→"R123":u16)  [unwired: 2 out]
            n215 = local write "R100"(w384) -> ()
            n216 = local write "R111"(w381) -> ()
            n217 = local write "R113"(w379) -> ()
            n218 = local write "R118"(w377) -> ()
          }
          frame "多个写入" {
            n219 = Unbundle By Name(w407) -> ("数据"=w406:variant)
            n220 = Variant To Data(type=T15 {"starting address"=0, "holding register values"=[]}, Variant=w406) -> (data=w404:T15)  [unwired: 1 in, 1 out]
            n221 = Unbundle By Name(w404) -> ("starting address"=w403:u16, "holding register values"=w402:u16[])
            n222 = call <vilib>:"Write Multiple Registers.vi"("error in (no error)"=w410, "values"=w402, "starting address"=w403, "MB session in"=w411) -> ("error out"=w409:errorcluster, "MB session out"=w408:refnum<class "MB_Master.lvclass">)  [unwired: 6 in]
          }
          frame "单个写入" {
            n223 = Unbundle By Name(w417) -> ("数据"=w416:variant)
            n224 = Variant To Data(type=T16 {"starting address"=0, "holding register value"=0}, Variant=w416) -> (data=w414:T16)  [unwired: 1 in, 1 out]
            n225 = Unbundle By Name(w414) -> ("starting address"=w413:u16, "holding register value"=w412:u16)
            n226 = call <vilib>:"Write Single Register.vi"("error in (no error)"=w420, "value"=w412, "address"=w413, "MB session in"=w421) -> ("error out"=w419:errorcluster, "MB session out"=w418:refnum<class "MB_Master.lvclass">)  [unwired: 6 in]
          }
          frame "线圈写入" {
            n227 = Unbundle By Name(w427) -> ("数据"=w426:variant)
            n228 = Variant To Data(type=T17 {"starting address"=0, "coil values"=[]}, Variant=w426) -> (data=w424:T17)  [unwired: 1 in, 1 out]
            n229 = Unbundle By Name(w424) -> ("starting address"=w423:u16, "coil values"=w422:bool[])
            n230 = call <vilib>:"Write Multiple Coils.vi"("error in (no error)"=w430, "values"=w422, "starting address"=w423, "MB session in"=w431) -> ("error out"=w429:errorcluster, "MB session out"=w428:refnum<class "MB_Master.lvclass">)  [unwired: 6 in]
          }
          frame "shutdown" {
            n231 = call <vilib>:"Write Single Register.vi"("error in (no error)"=w437, "value"=u16 0, "address"=u16 4047, "MB session in"=w441) -> ("error out"=w436:errorcluster, "MB session out"=w440:refnum<class "MB_Master.lvclass">)  [unwired: 6 in]
            n232 = call-dynamic "Close Session.vi"("error in (no error)"=w436, "MB session in"=w440) -> ("error out"=w442:errorcluster)  [unwired: 9 in]
            n233 = call "文件对话框"("start path"=path "D:/SRC") -> ("selected path"=w435:path, "cancelled"=w433:bool)  [unwired: 11 in, 2 out]
            n234 = call <vilib>:"Clear Errors.vi"("error in (no error)"=w442) -> ("error out"=w432:errorcluster)  [unwired: 5 in, 1 out]
            n235 = case shown="假" w433 {
              tunnel: w435 -> [w448 _]
              tunnel: w432 -> [_ _]
              frame False {
                n236 = Path To String(path=w448) -> (string=w445:string)
                n237 = Format Into String(format string="  - \"%s\"" ("格式字符串"), initial string="\"C:\\Program Files\\Fatek\\WinProladder\\WProlad.exe\"" ("command line"), w445) -> (resulting string=w446:string)  [unwired: 1 in, 1 out]
                n238 = call <vilib>:"System Exec.vi"("command line"=w446) -> ("error out"=w449:errorcluster)  [unwired: 7 in, 3 out]
                n239 = case shown="错误" w449 {
                  tunnel: w445 -> [_ w452]
                  frame No Error {
                  }
                  frame Error {
                    n240 = Format Into String(format string="  - \"%s\"" ("格式字符串"), initial string="\"C:\\Program Files (x86)\\Fatek\\WinProladder\\WProlad.exe\"" ("command line"), w452) -> (resulting string=w450:string)  [unwired: 1 in, 1 out]
                    n241 = call <vilib>:"System Exec.vi"("command line"=w450) -> ()  [unwired: 7 in, 4 out]
                  }
                }
              }
              frame True {
              }
            }
          }
        }
      }
      frame Error {
        n242 = Unbundle By Name(w458) -> ("code"=w460:i32)
        n243 = case shown="-1073807343" w460 {
          tunnel: w459 -> [w462 w466]
          tunnel: w458 -> [w461 w468]
          tunnel: [w461 w467] -> w456
          tunnel: [w462 w466] -> w457
          tunnel: w454 -> [_ w465]
          frame Default {
          }
          frame -1073807343 {
            n244 = Flush Queue(queue=w465) -> (queue out=w464:refnum<queue>)  [unwired: 1 in, 2 out]
            n245 = call-dynamic "Close Session.vi"("error in (no error)"=w468, "MB session in"=w466) -> ("error out"=w467:errorcluster)  [unwired: 9 in]
            n246 = disable-structure shown="禁用" {
              disable-tunnel: w464 -> [w469 _]
              frame Disabled {
                n247 = Enqueue Element At Opposite End(queue=w469, element=cluster{"命令":string, "数据":variant} {"命令"="init", "数据"=variant} ("元素")) -> ()  [unwired: 2 in, 3 out]
              }
              frame Enabled {
              }
            }
            n248 = Wait (ms)(milliseconds to wait=u32 2000 ("等待时间（毫秒）")) -> ()  [unwired: 1 out]
          }
        }
        n249 = call <vilib>:"Clear Errors.vi"("error in (no error)"=w456) -> ("error out"=w455:errorcluster)  [unwired: 5 in, 1 out]
      }
    }
    n250 = Unbundle By Name(w239) -> ("status"=→"通讯故障":bool)
  }
  n251 = property on="多列列表框" class="MCListbox (严格)"("ItemNames"=string[][] [["待机"], ["初始化"], ["水样润洗"], ["一级水样池进样"], ["沉淀"], ["二级水样池进样"], ["配水"], ["反冲洗"], ["采样池储水"], ["结束"]] ("项名")) -> ()  [unwired: 2 in, 2 out]
  n252 = call-dynamic "Close Session.vi"("error in (no error)"=w5, "MB session in"=w4) -> ()  [unwired: 9 in, 1 out]
